vi "MainController5.vi"() -> ()   [LabVIEW 2014]
doc: "The top-level MainController VI for the RCM Control Stack application.\n\n\nMike Schultz (mschultz11711@gmail.com)"
uses:
  SRV VIs/SubVIs/SRV_Response Data Type.ctl
  SRV VIs/Motors/Motors Config/SRV_Motor Control Button Icons_TRUE.ctl
  SRV VIs/Motors/Motors Config/SRV_Motor Control Button Icons_FALSE.ctl
  SRV VIs/ImageProcessing/QR Code Detection Radio Buttons.ctl
  SRV VIs/SubVIs/SRV_SRV_Loops Notifier Methods.ctl
  SRV VIs/SRV_Main Controller Local Data.ctl
  SRV VIs/Motors/Motors Config/SRV_Motor Control Button Config.ctl
  SRV VIs/Motors/Motors Config/SRV_Motor Legos-Servo.ctl
  SRV VIs/Motors/Motors Config/SRV_Motor Control Commands Cluster.ctl
  SRV VIs/Motors/Motors Config/SRV_Motor Control Command Config.ctl
  SRV VIs/SubVIs/SRV_Streaming States.ctl
  SRV VIs/SubVIs/SRV_Streaming State.ctl
  SRV VIs/PacketMode/SRV_PM_Packet Mode Style.ctl
  SRV VIs/Support/SRV_Command-Data Queue Data Type.ctl
  SRV VIs/PacketMode/SRV_PM_Packet.ctl
  SRV VIs/Motors/SRV_Button Event Data.ctl
  SRV VIs/SubVIs/SRV_Streaming Modes.ctl
  <vilib>/Utility/miscctls.llb/LVBoundsTypeDef.ctl
  SRV VIs/ImageProcessing/QT_Image.ctl
  SRV VIs/SubVIs/SRV_Number of IMJ Requests Methods.ctl
  SRV VIs/SubVIs/SRVGlobals.vi
panel:
  in  "Window Enabled?":bool=TRUE
  out "Text.Scroll Position":u32
  in  "button E5":bool
  out "true E5":T1
  out "false E5":T2
  in  "button E4":bool
  out "true E4":T1
  out "false E4":T2
  in  "button E3":bool
  out "true E3":T1
  out "false E3":T2
  in  "button E1":bool
  out "true E1":T1
  out "false E1":T2
  in  "button E2":bool
  out "true E2":T1
  out "false E2":T2
  in  "button E7":bool
  out "true E7":T1
  out "false E7":T2
  in  "button E6":bool
  out "true E6":T1
  out "false E6":T2
  in  "button D7":bool
  out "true D7":T1
  out "false D7":T2
  in  "button A7":bool
  out "true A7":T1
  out "false A7":T2
  in  "button C7":bool
  out "true C7":T1
  out "false C7":T2
  in  "button B7":bool
  out "true B7":T1
  out "false B7":T2
  in  "button D6":bool
  out "true D6":T1
  out "false D6":T2
  in  "button A6":bool
  out "true A6":T1
  out "false A6":T2
  in  "button C6":bool
  out "true C6":T1
  out "false C6":T2
  in  "button B6":bool
  out "true B6":T1
  out "false B6":T2
  in  "button D5":bool
  out "true D5":T1
  out "false D5":T2
  in  "button A5":bool
  out "true A5":T1
  out "false A5":T2
  in  "button C5":bool
  out "true C5":T1
  out "false C5":T2
  in  "button B5":bool
  out "true B5":T1
  out "false B5":T2
  in  "button D4":bool
  out "true D4":T1
  out "false D4":T2
  in  "button A4":bool
  out "true A4":T1
  out "false A4":T2
  in  "button C4":bool
  out "true C4":T1
  out "false C4":T2
  in  "button B4":bool
  out "true B4":T1
  out "false B4":T2
  in  "button D3":bool
  out "true D3":T1
  out "false D3":T2
  in  "button A3":bool
  out "true A3":T1
  out "false A3":T2
  in  "button C3":bool
  out "true C3":T1
  out "false C3":T2
  in  "button B3":bool
  out "true B3":T1
  out "false B3":T2
  in  "button D2":bool
  out "true D2":T1
  out "false D2":T2
  in  "button A2":bool
  out "true A2":T1
  out "false A2":T2
  in  "button C2":bool
  out "true C2":T1
  out "false C2":T2
  in  "button B2":bool
  out "true B2":T1
  out "false B2":T2
  in  "Expand-Collapse":bool
  in  "button D1":bool
  out "true D1":T1
  out "false D1":T2
  in  "button A1":bool
  out "true A1":T1
  out "false A1":T2
  in  "button C1":bool
  out "true C1":T1
  out "false C1":T2
  in  "button B1":bool
  out "true B1":T1
  out "false B1":T2
  out "Overflow Indicator":bool
  out "ms Diff 3":u32
  out "ms Diff 2":u32
  out "ms Diff parse":u32
  out "ms Diff ##IMJ":u32
  out "ms Diff DQ":u32
  out "ms Diff":u32
  out "Response Data Type":T3=enum."No Data"
  out "i4":i32
  in  "Show Image":bool
  out "InPico State Change":bool
  in  "clear":bool
  out "Replies":string
  out "Number of IMJ Requests":i32
  out "XModem Replies":string[](array[string])
  out "i1":i32
  out "i2":i32
  out "Status":string
  out "The image":picture caption="new picture"
  out "IP Address":string
  out "In Pico":bool
  out "connected?":bool
  in  "Tab Control":T4(tab)=enum."Camera View"
  in  "Send Text":bool
  in  "ESC":bool
  in  "Direct Command to Send":string
  in  "Run CCode":bool
  in  "View Code":bool
  in  "Upload CCode":bool
  in  "C Code":string="int x,y,z;\nfor (x = 0; x < 2; x++) \n  {  \n    for (y = 0; y < 3; y++)\n       {       \n         for (z = 0; z < 2; z++)\n           {\n             printf(\"%d %d %d\\n\", x,y,z);   \n           }\n        } \n   }\nexit(1);"
  in  "load Text":bool
  in  "QR Code Detection":T5
  in  "Movie":bool
  in  "Camera":bool
  out "Cover":bool
  in  "Images Directory Path":path=path "C:/RCM_Images"
  out "YUV_SRV":cluster{"Y":sgl, "U":sgl, "V":sgl}
  in  "Plan":T6(radio)
  out "YUV_Calc":cluster{"Y":sgl, "U":sgl, "V":sgl}
  in  "Plan 2":T7(radio)
  in  "Plan 3":enum32{"Nothing", "Differencing"}(radio)
  in  "Plan 4":T8(radio)
  in  "Color to Send":string
  in  "Send Color":bool
  in  "vc Bins":T9(ring)=enum."Bin 2"
  in  "Show  Overlay":bool
  in  "Flip Image":bool
  in  "vz Bins":T10(ring)=enum."4 levels of U and 4 levels of V"
  in  "Threshold":i8(slide)=4 scale=1.0..9.0
  in  "firmware":path
  in  "Upload":bool
  in  "Version":bool
  in  "Edit Sensors Config":bool
  in  "Edit System Config":bool
  out "System Config":string
  in  "Edit Motors Config":bool
  in  "stop":bool
  # "Communication"
  # "Debug indicators below.\nA developer just needs to enlarge the decoration to include these at debug time."
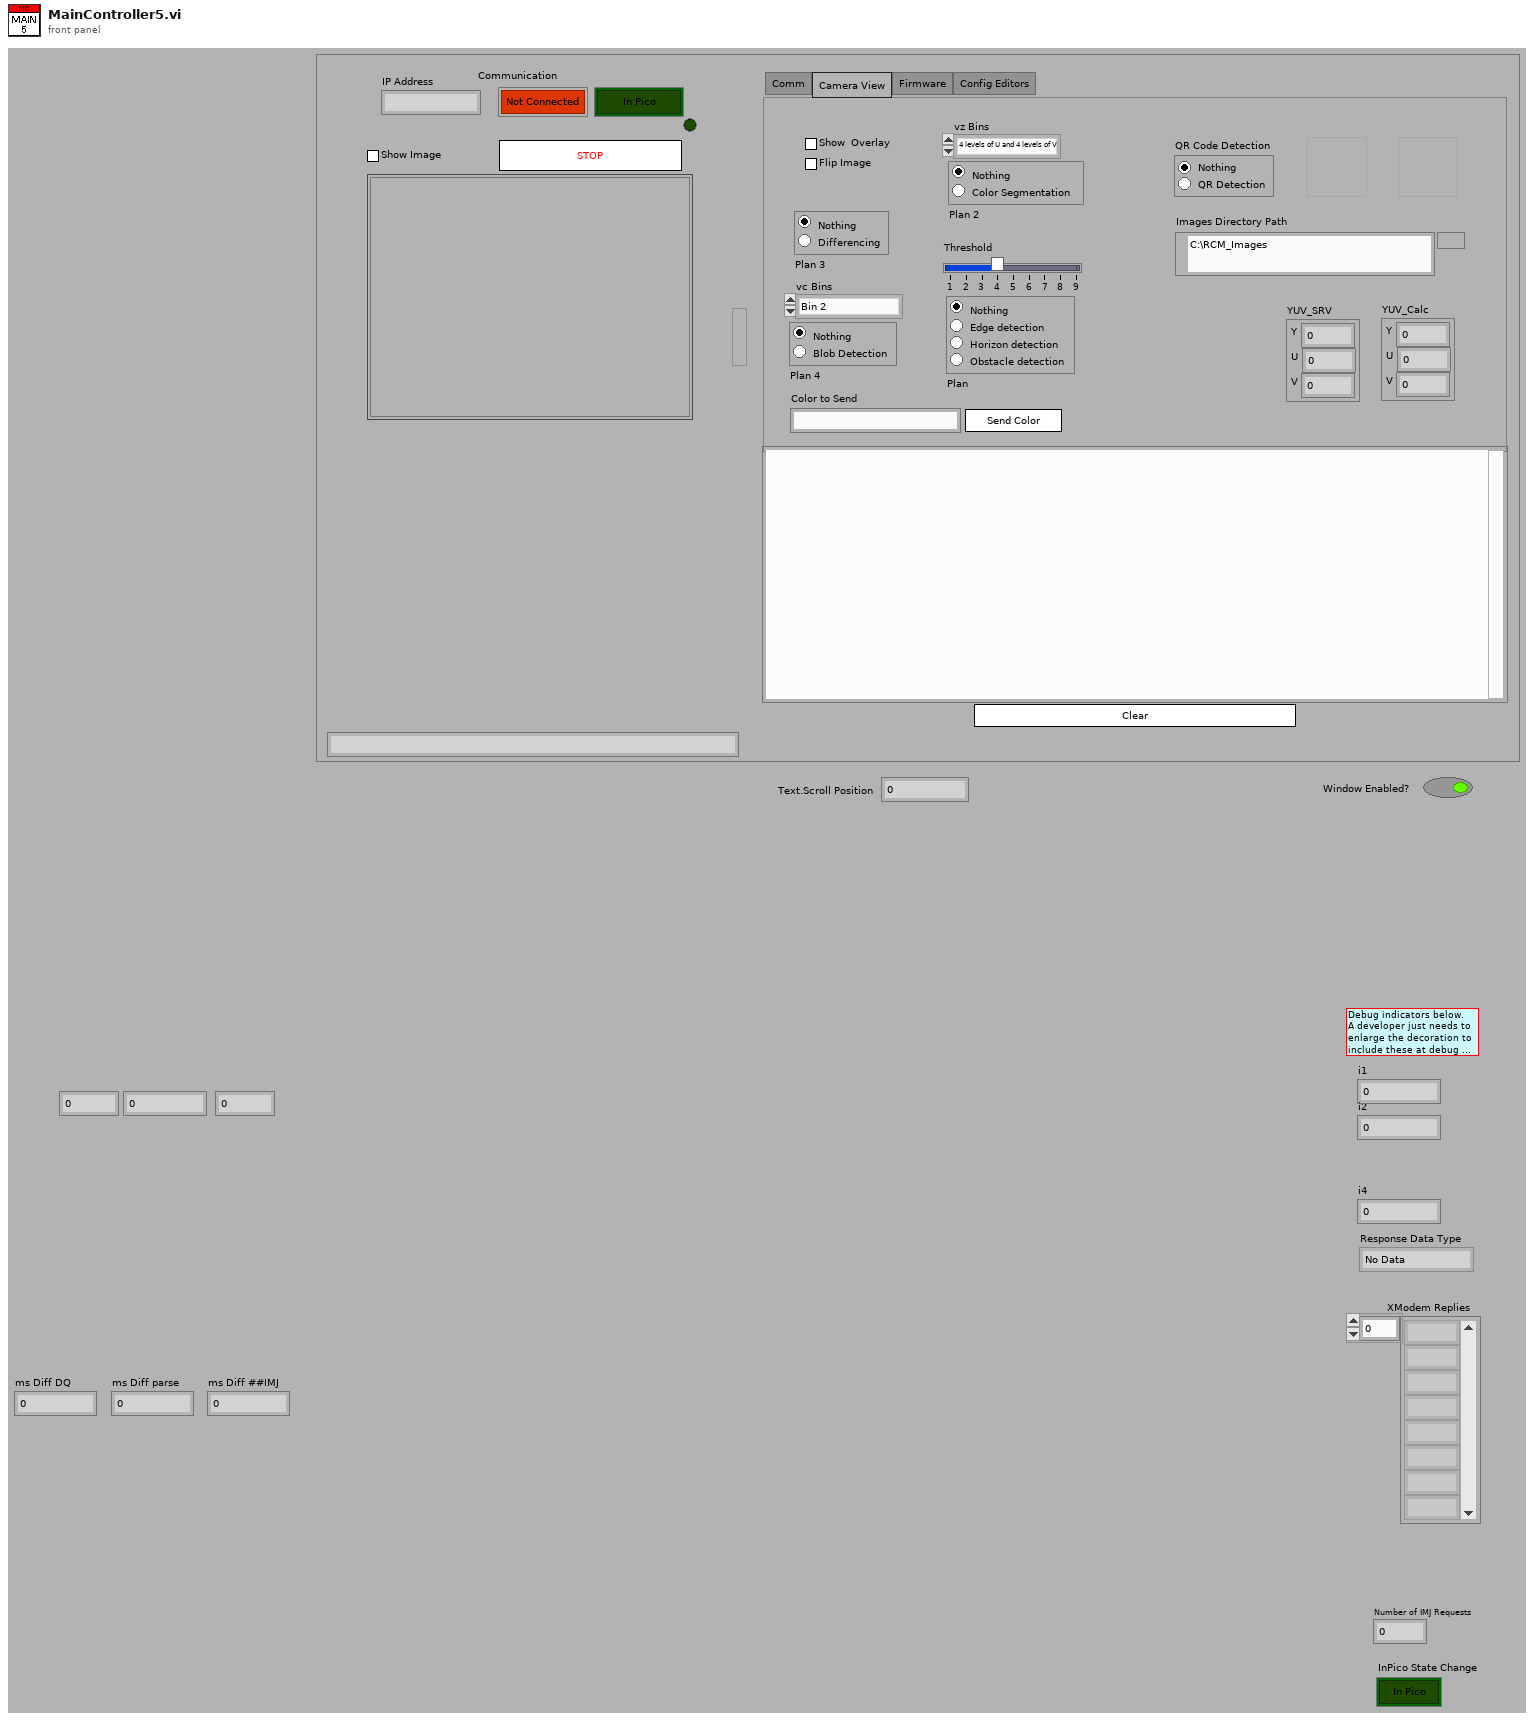
[diagram p1: front panel]
types:
  T1 = typedef "SRV_Motor Control Button Icons_TRUE.ctl" = u16
  T2 = typedef "SRV_Motor Control Button Icons_FALSE.ctl" = u16
  T3 = typedef "SRV_Response Data Type.ctl" = enum16{"Undefined Data", "##IMJ", "#B", "Leaving PicoC", "##vp", "##zZ", "##g:7", "##N$B", "##N$b", "##i$l", "##i$L", "##i$N", "##&NP,", "##&R,", "No Data"}
  T4 = enum32{"Comm", "Camera View", "Firmware", "Config Editors"}
  T5 = typedef "QR Code Detection Radio Buttons.ctl" = enum32{"Nothing", "QR Detection"}
  T6 = enum32{"Nothing", "Differencing", "Color Segmentation", "Edge detection", "Horizon detection", "Obstacle detection"}
  T7 = enum32{"Nothing", "Differencing", "Color Segmentation"}
  T8 = enum32{"Nothing", "Differencing", "Color Segmentation", "Edge detection", "Horizon detection", "Obstacle detection", "Blob Detection"}
  T9 = enum16{"Bin 0", "Bin 1", "Bin 2", "Bin 3", "Bin 4", "Bin 5", "Bin 6", "Bin 7", "Bin 9", "Bin 8", "Bin 10", "Bin 11", "Bin 12", "Bin 13", "Bin 14", "Bin 15"}
  T10 = enum16{"Zero all", "4 levels of Y, 2 levels of U, 2 levels of V", "4 levels of U and 4 levels of V", "even distribution across U and V", "16 grayscale levels"}
  T11 = typedef "SRV_Main Controller Local Data.ctl" = cluster{"user event":refnum<user-event>, "SRV":refnum<k5>, "Replies":refnum<vi>, "Status":refnum<vi>, "false refs":refnum<vi>[], "true refs":refnum<vi>[], "Motor Control Config":T12[], "Default Config Dir":path, "System Config Name":string, "Cached Streaming States":T16, "Main Controller ref":refnum<vi>, "Sensor View ref":refnum<vi>, "VISTA or Later?":bool, "button refs":refnum<vi>[]}
  T12 = typedef "SRV_Motor Control Button Config.ctl" = cluster{"Button Name":string, "Button Label":string, "Motor Type":T13, "Press Cmds":T14, "Release Cmds":T14, "Icon":T2}
  T13 = typedef "SRV_Motor Legos-Servo.ctl" = enum16{"Servo", "Legos", "Shared Var"}
  T14 = typedef "SRV_Motor Control Commands Cluster.ctl" = cluster{"Motor Control Commands Array":T15[]}
  T15 = typedef "SRV_Motor Control Command Config.ctl" = cluster{"I2C Address":u8, "Register":u8, "Value":u8, "Active":bool}
  T16 = typedef "SRV_Streaming States.ctl" = cluster{"Video":T17, "Sensors":T17}
  T17 = typedef "SRV_Streaming State.ctl" = cluster{"Enabled":bool, "Data":string}
  T18 = typedef "SRV_SRV_Loops Notifier Methods.ctl" = enum16{"Wait on Notification", "Send Notification", "Release Notifier"}
  T19 = typedef "SRV_PM_Packet.ctl" = cluster{"Packet Data":u8[], "Header Complete?":bool, "Complete?":bool, "Checksum OK?":bool, "Error?":bool}
  T20 = enum8{"Enabled", "Disabled", "Disabled and Grayed Out"}
  T21 = typedef "SRV_Command-Data Queue Data Type.ctl" = cluster{"Command":string, "Data":variant}
  T22 = typedef "SRV_PM_Packet Mode Style.ctl" = enum16{"Old", "New PM"}
  T23 = typedef "Semaphore RefNum" = refnum<k1>
  T24 = typedef "SRV_Button Event Data.ctl" = cluster{"Button NewVal":bool, "Button Index":i32}
  T25 = enum16{"Disable", "Frame Differencing", "Color Segmentation", "Edge Detection", "Horizon detection", "Obstacle detection", "Blob Detection", "Stereo processing"}
  T26 = typedef "SRV_Streaming Modes.ctl" = enum16{"Video", "Sensors"}
  T27 = typedef "LVBoundsTypeDef.ctl" = cluster{"Width":u32, "Height":u32}
  T28 = typedef "SRV_Number of IMJ Requests Methods.ctl" = enum16{"Read", "Increment", "Decrement", "Reset", "Close"}
  T29 = typedef "SRV_System Config.ctl" = cluster{"SRV IP Address":string, "Video Stream Rate Period (ms)":u32, "Enable Diagnostic Log":bool, "Watchdog 1 Config":T30, "Watchdog 2 Config":T30, "Sensor Window Filepath":path}
  T30 = typedef "SRV_Watchdog Config Cluster.ctl" = cluster{"Watchdog Name":string, "Watchdog Period (s)":dbl, "Watchdog Command":T15}
  T31 = typedef "QT_Image.ctl" = cluster{"Witdh":i32, "Height":i32, "Depth":i32, "data":u8[], "Compressed data":u8[], "Color table":u32[], "Duration":i32, "Options":i32, "Timestamp":i32, "ID":i32, "Reserved":i32, "Dialogs":u32}
  T32 = typedef "LVMouseTypeDef.ctl" = cluster{"Mouse Position":cluster{"X":i32, "Y":i32}, "Mouse Modifiers":cluster{"Button Down":bool, "Shift Mod":bool, "Menu Mod":bool, "Option Mod":bool}}
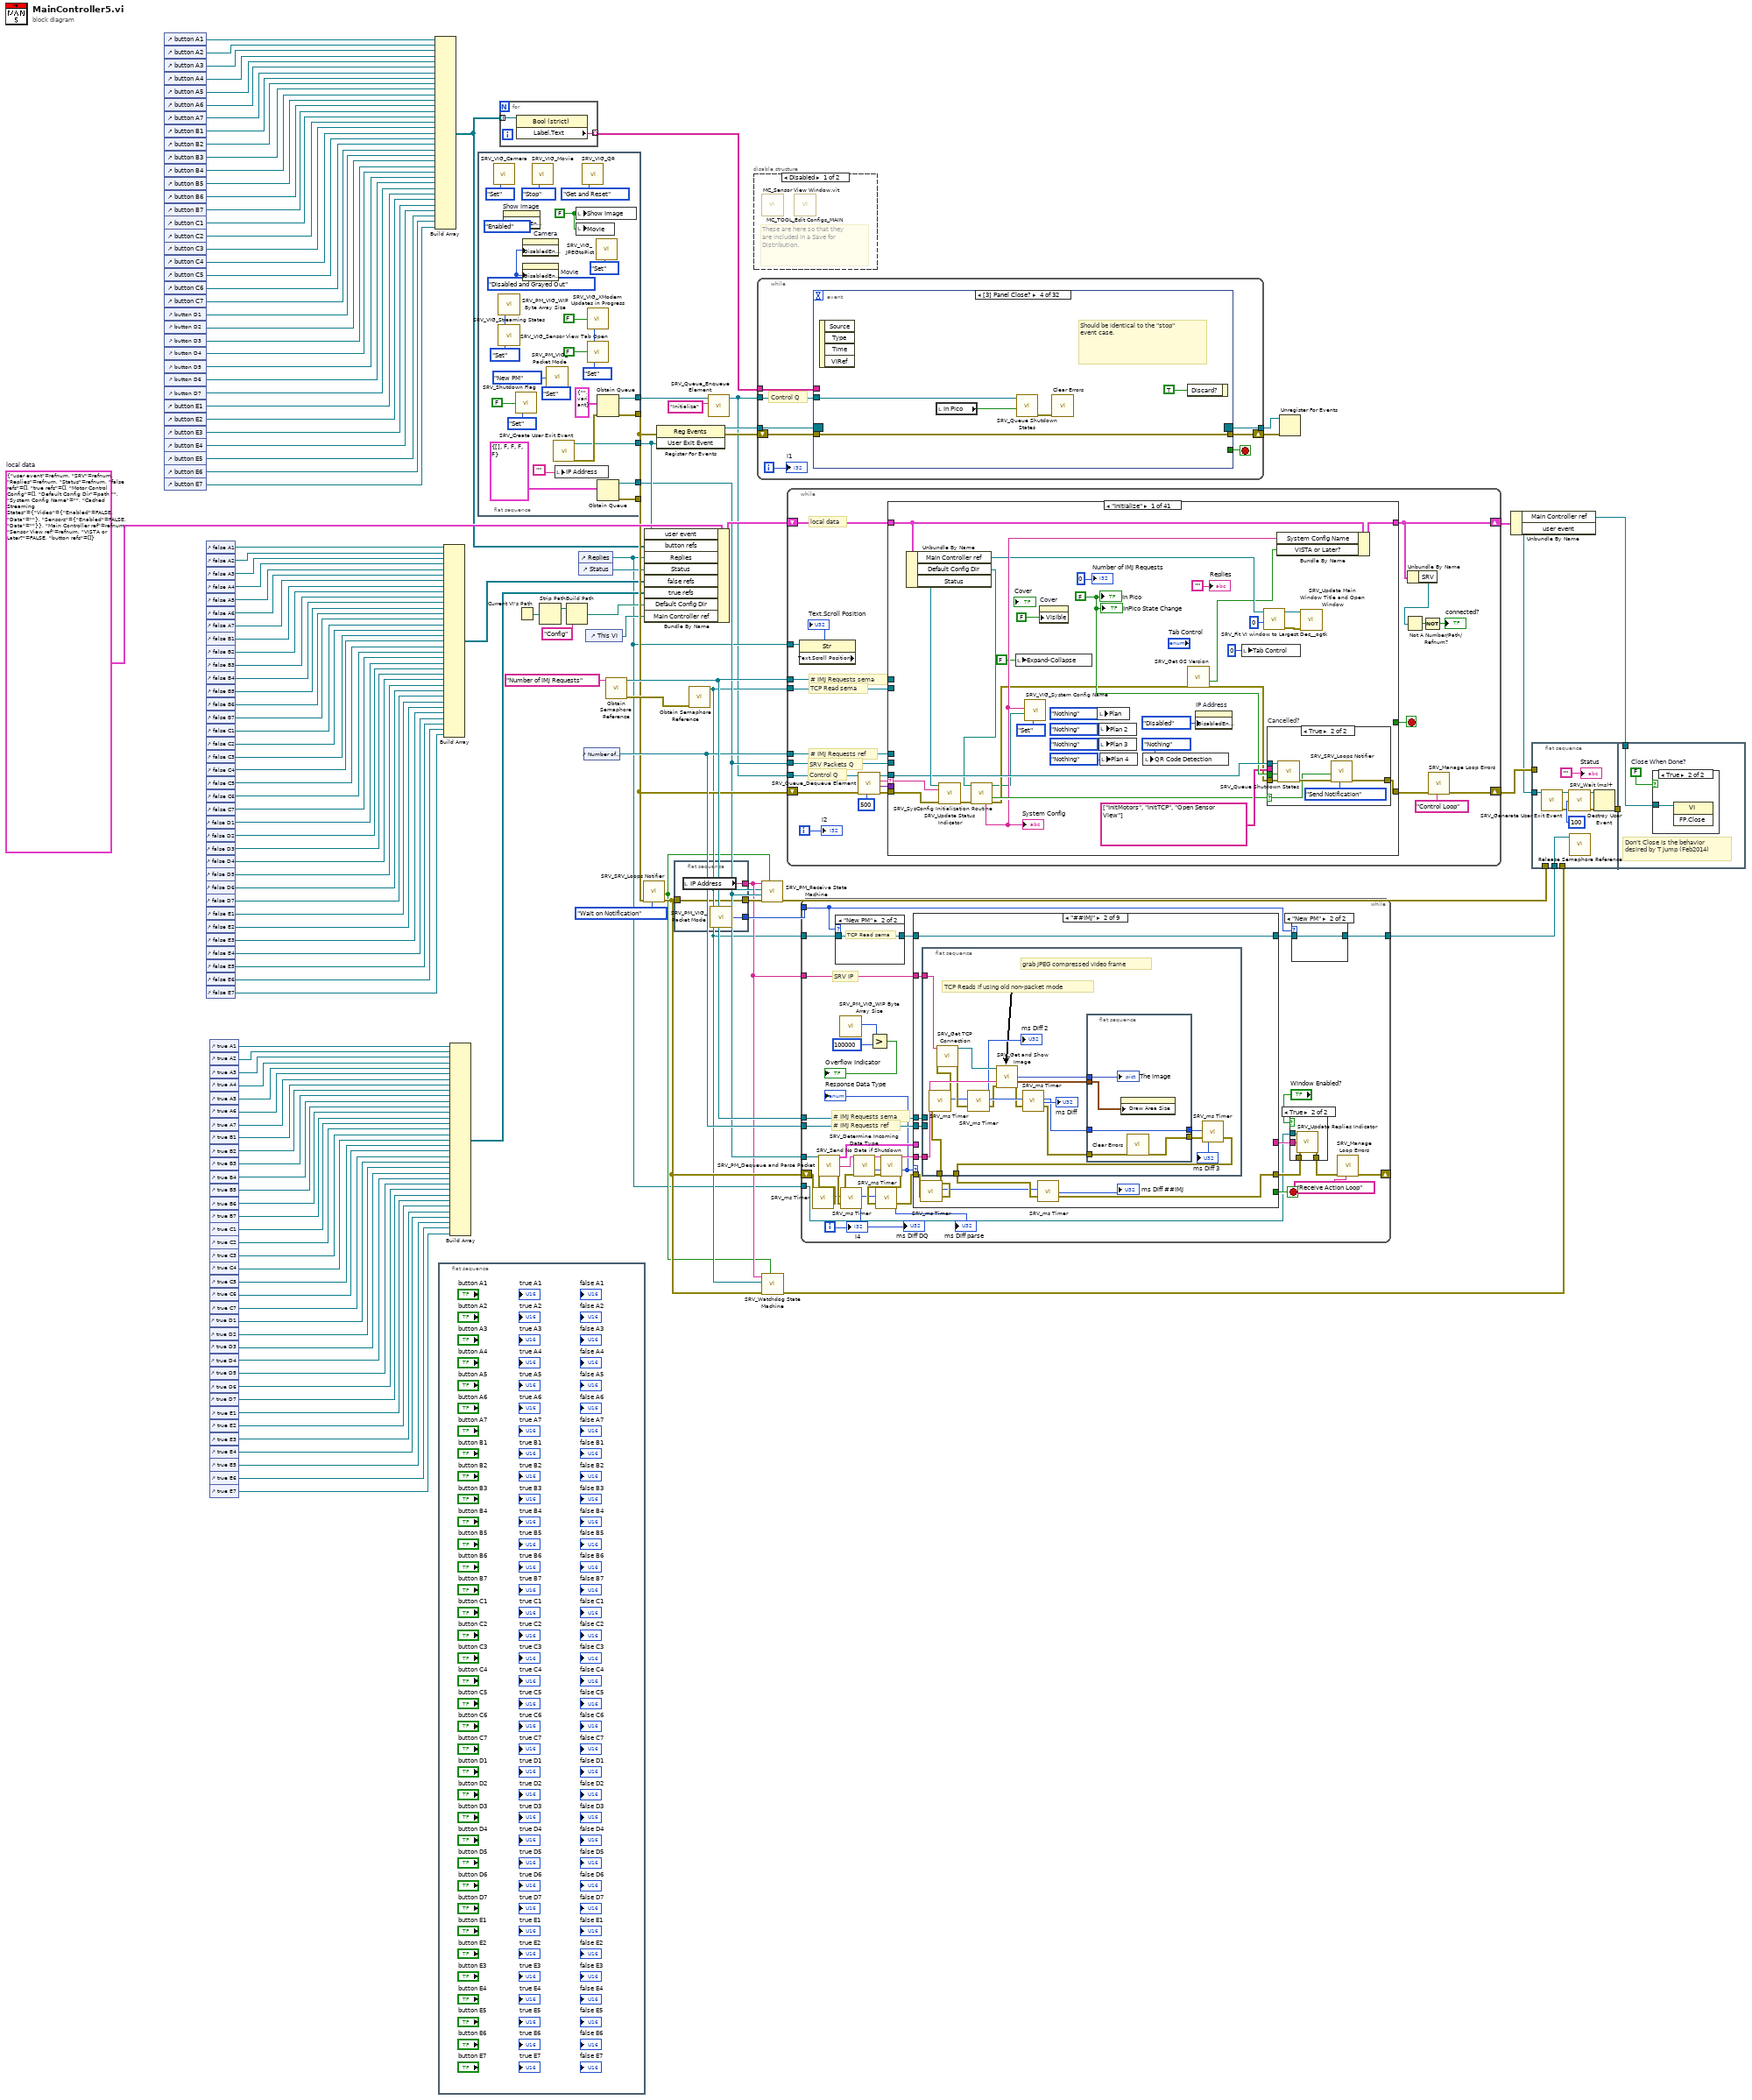
[diagram p0: block diagram]
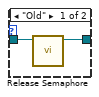
[diagram p5: hidden frame]
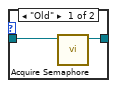
[diagram p6: hidden frame]
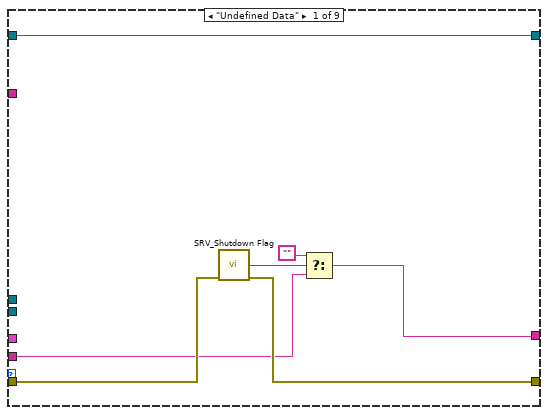
[diagram p7: hidden frame]
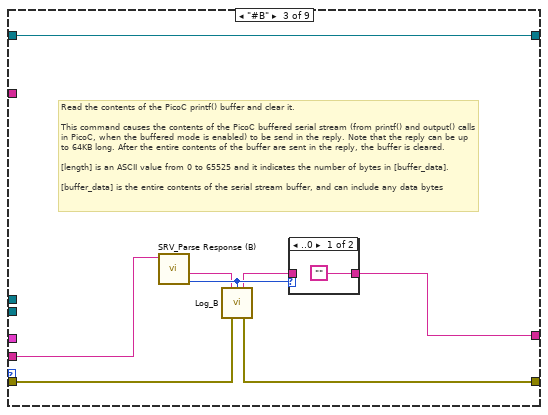
[diagram p8: hidden frame]
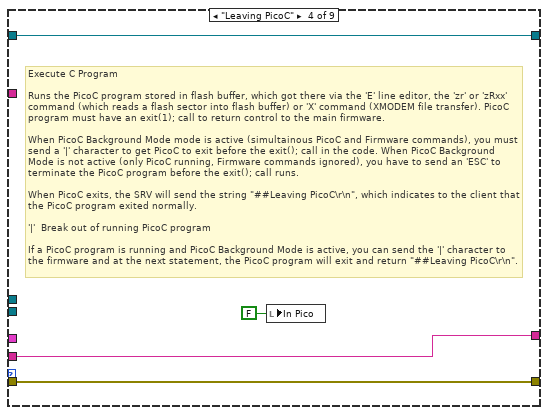
[diagram p10: hidden frame]
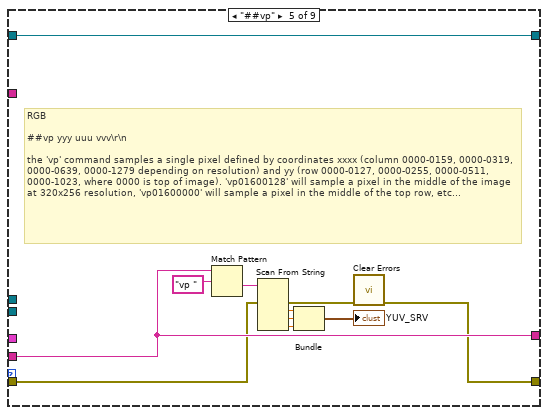
[diagram p11: hidden frame]
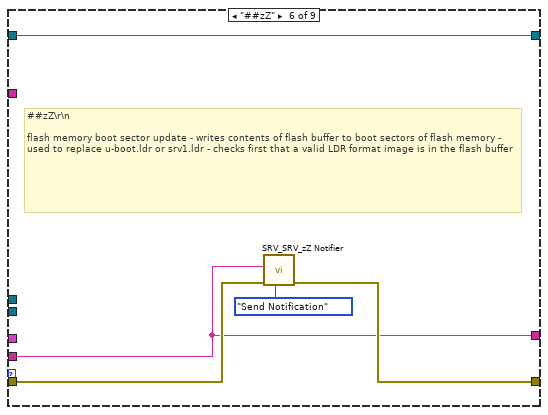
[diagram p12: hidden frame]
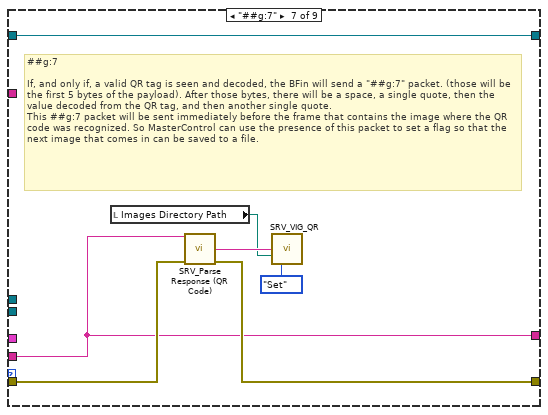
[diagram p13: hidden frame]
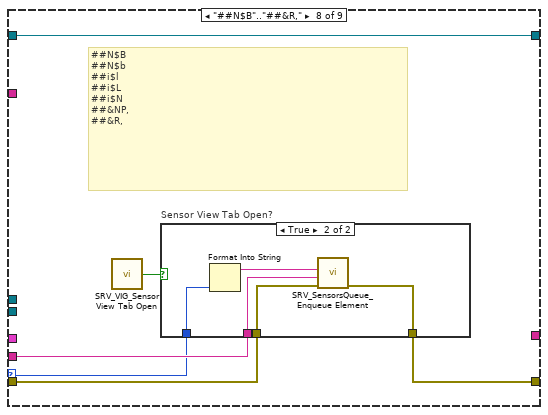
[diagram p14: hidden frame]
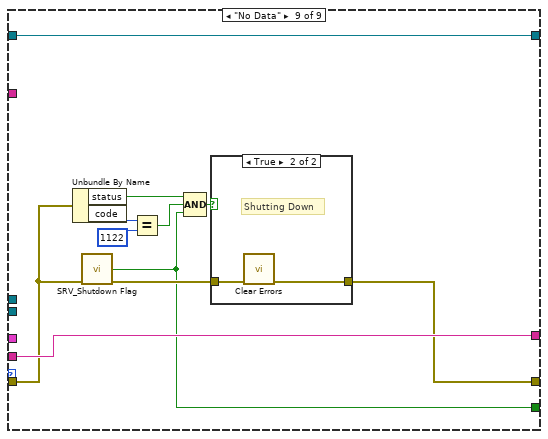
[diagram p16: hidden frame]
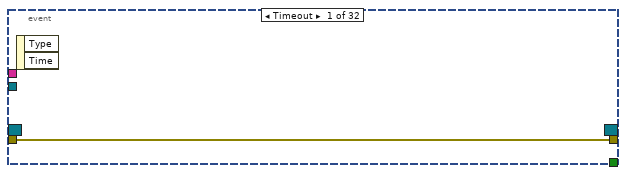
[diagram p18: hidden frame]
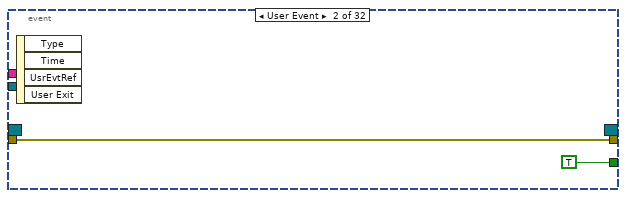
[diagram p19: hidden frame]
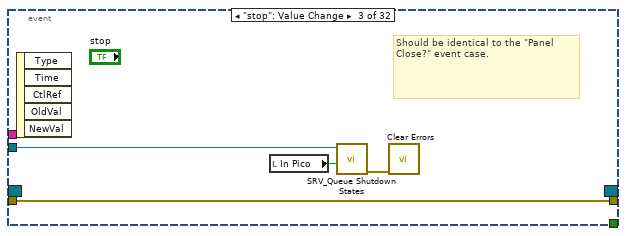
[diagram p20: hidden frame]
diagram:
  w136 = T11 {"user event"=refnum, "SRV"=refnum, "Replies"=refnum, "Status"=refnum, "false refs"=[], "true refs"=[], "Motor Control Config"=[], "Default Config Dir"=path "", "System Config Name"="", "Cached Streaming States"={"Video"={"Enabled"=FALSE, "Data"=""}, "Sensors"={"Enabled"=FALSE, "Data"=""}}, "Main Controller ref"=refnum, "Sensor View ref"=refnum, "VISTA or Later?"=FALSE, "button refs"=[]}  # local data
  n1 = control-ref of="button A1"() -> (w108:refnum<vi>)
  n2 = control-ref of="button A2"() -> (w107:refnum<vi>)
  n3 = control-ref of="button A3"() -> (w106:refnum<vi>)
  n4 = control-ref of="button A4"() -> (w105:refnum<vi>)
  n5 = control-ref of="button A5"() -> (w104:refnum<vi>)
  n6 = control-ref of="button A6"() -> (w103:refnum<vi>)
  n7 = control-ref of="button A7"() -> (w102:refnum<vi>)
  n8 = control-ref of="button B1"() -> (w101:refnum<vi>)
  n9 = control-ref of="button B2"() -> (w100:refnum<vi>)
  n10 = control-ref of="button B3"() -> (w99:refnum<vi>)
  n11 = control-ref of="button B4"() -> (w98:refnum<vi>)
  n12 = control-ref of="button B5"() -> (w97:refnum<vi>)
  n13 = control-ref of="button B6"() -> (w96:refnum<vi>)
  n14 = control-ref of="button B7"() -> (w95:refnum<vi>)
  n15 = control-ref of="button C1"() -> (w94:refnum<vi>)
  n16 = control-ref of="button C2"() -> (w93:refnum<vi>)
  n17 = control-ref of="button C3"() -> (w92:refnum<vi>)
  n18 = control-ref of="button C4"() -> (w91:refnum<vi>)
  n19 = control-ref of="button C5"() -> (w90:refnum<vi>)
  n20 = control-ref of="button C6"() -> (w89:refnum<vi>)
  n21 = control-ref of="button C7"() -> (w88:refnum<vi>)
  n22 = control-ref of="button D1"() -> (w87:refnum<vi>)
  n23 = control-ref of="button D2"() -> (w86:refnum<vi>)
  n24 = control-ref of="button D3"() -> (w85:refnum<vi>)
  n25 = control-ref of="button D4"() -> (w84:refnum<vi>)
  n26 = control-ref of="button D5"() -> (w83:refnum<vi>)
  n27 = control-ref of="button D6"() -> (w82:refnum<vi>)
  n28 = control-ref of="button D7"() -> (w81:refnum<vi>)
  n29 = control-ref of="button E1"() -> (w23:refnum<vi>)
  n30 = control-ref of="button E2"() -> (w22:refnum<vi>)
  n31 = control-ref of="button E3"() -> (w21:refnum<vi>)
  n32 = control-ref of="button E4"() -> (w20:refnum<vi>)
  n33 = control-ref of="button E5"() -> (w19:refnum<vi>)
  n34 = control-ref of="button E6"() -> (w18:refnum<vi>)
  n35 = control-ref of="button E7"() -> (w17:refnum<vi>)
  n36 = control-ref of="false A1"() -> (w52:refnum<vi>)
  n37 = control-ref of="false A2"() -> (w51:refnum<vi>)
  n38 = control-ref of="false A3"() -> (w50:refnum<vi>)
  n39 = control-ref of="false A4"() -> (w49:refnum<vi>)
  n40 = control-ref of="false A5"() -> (w48:refnum<vi>)
  n41 = control-ref of="false A6"() -> (w47:refnum<vi>)
  n42 = control-ref of="false A7"() -> (w46:refnum<vi>)
  n43 = control-ref of="false B1"() -> (w45:refnum<vi>)
  n44 = control-ref of="false B2"() -> (w44:refnum<vi>)
  n45 = control-ref of="false B3"() -> (w43:refnum<vi>)
  n46 = control-ref of="false B4"() -> (w42:refnum<vi>)
  n47 = control-ref of="false B5"() -> (w41:refnum<vi>)
  n48 = control-ref of="false B6"() -> (w40:refnum<vi>)
  n49 = control-ref of="false B7"() -> (w39:refnum<vi>)
  n50 = control-ref of="false C1"() -> (w38:refnum<vi>)
  n51 = control-ref of="false C2"() -> (w37:refnum<vi>)
  n52 = control-ref of="false C3"() -> (w36:refnum<vi>)
  n53 = control-ref of="false C4"() -> (w35:refnum<vi>)
  n54 = control-ref of="false C5"() -> (w34:refnum<vi>)
  n55 = control-ref of="false C6"() -> (w33:refnum<vi>)
  n56 = control-ref of="false C7"() -> (w32:refnum<vi>)
  n57 = control-ref of="false D1"() -> (w31:refnum<vi>)
  n58 = control-ref of="false D2"() -> (w30:refnum<vi>)
  n59 = control-ref of="false D3"() -> (w29:refnum<vi>)
  n60 = control-ref of="false D4"() -> (w28:refnum<vi>)
  n61 = control-ref of="false D5"() -> (w27:refnum<vi>)
  n62 = control-ref of="false D6"() -> (w26:refnum<vi>)
  n63 = control-ref of="false D7"() -> (w25:refnum<vi>)
  n64 = control-ref of="false E1"() -> (w9:refnum<vi>)
  n65 = control-ref of="false E2"() -> (w8:refnum<vi>)
  n66 = control-ref of="false E3"() -> (w7:refnum<vi>)
  n67 = control-ref of="false E4"() -> (w6:refnum<vi>)
  n68 = control-ref of="false E5"() -> (w5:refnum<vi>)
  n69 = control-ref of="false E6"() -> (w4:refnum<vi>)
  n70 = control-ref of="false E7"() -> (w3:refnum<vi>)
  n71 = control-ref of="true A1"() -> (w80:refnum<vi>)
  n72 = control-ref of="true A2"() -> (w79:refnum<vi>)
  n73 = control-ref of="true A3"() -> (w78:refnum<vi>)
  n74 = control-ref of="true A4"() -> (w77:refnum<vi>)
  n75 = control-ref of="true A5"() -> (w76:refnum<vi>)
  n76 = control-ref of="true A6"() -> (w75:refnum<vi>)
  n77 = control-ref of="true A7"() -> (w74:refnum<vi>)
  n78 = control-ref of="true B1"() -> (w73:refnum<vi>)
  n79 = control-ref of="true B2"() -> (w72:refnum<vi>)
  n80 = control-ref of="true B3"() -> (w71:refnum<vi>)
  n81 = control-ref of="true B4"() -> (w70:refnum<vi>)
  n82 = control-ref of="true B5"() -> (w69:refnum<vi>)
  n83 = control-ref of="true B6"() -> (w68:refnum<vi>)
  n84 = control-ref of="true B7"() -> (w67:refnum<vi>)
  n85 = control-ref of="true C1"() -> (w66:refnum<vi>)
  n86 = control-ref of="true C2"() -> (w65:refnum<vi>)
  n87 = control-ref of="true C3"() -> (w64:refnum<vi>)
  n88 = control-ref of="true C4"() -> (w63:refnum<vi>)
  n89 = control-ref of="true C5"() -> (w62:refnum<vi>)
  n90 = control-ref of="true C6"() -> (w61:refnum<vi>)
  n91 = control-ref of="true C7"() -> (w60:refnum<vi>)
  n92 = control-ref of="true D1"() -> (w59:refnum<vi>)
  n93 = control-ref of="true D2"() -> (w58:refnum<vi>)
  n94 = control-ref of="true D3"() -> (w57:refnum<vi>)
  n95 = control-ref of="true D4"() -> (w56:refnum<vi>)
  n96 = control-ref of="true D5"() -> (w55:refnum<vi>)
  n97 = control-ref of="true D6"() -> (w54:refnum<vi>)
  n98 = control-ref of="true D7"() -> (w53:refnum<vi>)
  n99 = control-ref of="true E1"() -> (w16:refnum<vi>)
  n100 = control-ref of="true E2"() -> (w15:refnum<vi>)
  n101 = control-ref of="true E3"() -> (w14:refnum<vi>)
  n102 = control-ref of="true E4"() -> (w13:refnum<vi>)
  n103 = control-ref of="true E5"() -> (w12:refnum<vi>)
  n104 = control-ref of="true E6"() -> (w11:refnum<vi>)
  n105 = control-ref of="true E7"() -> (w10:refnum<vi>)
  n106 = Build Array(w108, w107, w106, w105, w104, w103, w102, w101, w100, w99, w98, w97, w96, w95, w94, w93, w92, w91, w90, w89, w88, w87, w86, w85, w84, w83, w82, w81, w23, w22, w21, w20, w19, w18, w17) -> (w24:refnum<vi>[])
  n107 = flat-sequence {
    frame #0 {
    }
  }
  n108 = Build Array(w52, w51, w50, w49, w48, w47, w46, w45, w44, w43, w42, w41, w40, w39, w38, w37, w36, w35, w34, w33, w32, w31, w30, w29, w28, w27, w26, w25, w9, w8, w7, w6, w5, w4, w3) -> (w124:refnum<vi>[])
  n109 = Build Array(w80, w79, w78, w77, w76, w75, w74, w73, w72, w71, w70, w69, w68, w67, w66, w65, w64, w63, w62, w61, w60, w59, w58, w57, w56, w55, w54, w53, w16, w15, w14, w13, w12, w11, w10) -> (w123:refnum<vi>[])
  n110 = flat-sequence {
    tunnel: [w165] -> w137
    tunnel: [w166] -> w132
    tunnel: [w163] -> w133
    tunnel: [w159] -> w116
    tunnel: [w158] -> _
    frame #0 {
      w152 = T20."Disabled and Grayed Out" ("Disabled")
      w155 = enum16{"Get", "Set"}."Set" ("Method (Get)")
      w156 = enum16{"Get", "Set"}."Set" ("Method (Get)")
      w153 = FALSE ("Show Image")
      n111 = call "SRV_VIG_Camera.vi"("Method (Get)"=enum16{"Get", "Set"}."Set") -> ()  [unwired: 13 in, 2 out]
      n112 = call "SRV_PM_VIG_WIP Byte Array Size.vi"("Method (Get)"=w156) -> ()  [unwired: 9 in, 2 out]
      n113 = call "SRV_VIG_Streaming States.vi"("Method (Get)"=w156) -> ()  [unwired: 14 in, 1 out]
      n114 = property on="Show Image" class="Bool (strict)"("DisabledEnum"=T20."Enabled" ("Disabled")) -> ()  [unwired: 2 in, 2 out]
      n115 = call "SRV_Shutdown Flag.vi"("Shutdown Flag"=FALSE, "Method (Get)"=enum16{"Get", "Set"}."Set") -> ()  [unwired: 12 in, 2 out]
      n116 = property on="Camera" class="Bool"("DisabledEnum"=w152) -> ()  [unwired: 2 in, 2 out]
      n117 = property on="Movie" class="Bool (strict)"("DisabledEnum"=w152) -> ()  [unwired: 2 in, 2 out]
      n118 = call "SRV_VIG_Movie.vi"("Method (Get)"=enum16{"Get", "Start", "Stop"}."Stop") -> ()  [unwired: 11 in, 4 out]
      n119 = call "SRV_PM_VIG_Packet Mode.vi"("Packet Mode Style"=SRV_PM_Packet_Mode_Style."New PM", "Method (Get)"=enum16{"Get", "Set"}."Set") -> ()  [unwired: 13 in, 1 out]
      n120 = call "SRV_Create User Exit Event.vi"() -> ("error out"=w164:errorcluster, "User Exit Event"=w163:refnum<user-event>)  [unwired: 10 in]
      n121 = local write "IP Address"("") -> ()
      n122 = local write "Show Image"(w153) -> ()
      n123 = local write "Movie"(w153) -> ()
      n124 = call "SRV_VIG_QR.vi"("Method (Get and Reset)"=enum16{"Get and Reset", "Set"}."Get and Reset") -> ()  [unwired: 11 in, 4 out]
      n125 = call "SRV_VIG_XModem Updates in Progress.vi"("XModem Updates in Progress"=FALSE, "Method (Get)"=w155) -> ()  [unwired: 12 in, 2 out]
      n126 = call "SRV_VIG_Sensor View Tab Open.vi"("Sensor View Tab Open"=FALSE, "Method (Get)"=w155) -> ()  [unwired: 12 in, 2 out]
      n127 = call "SRV_VIG_JPEGtoPict.vi"("Method (Get)"=enum16{"Get", "Set"}."Set") -> ()  [unwired: 9 in, 2 out]
      n128 = Obtain Queue(element data type=T21 {"Command"="", "Data"=variant} ("Queue Data Type"), error in (no error)=w164) -> (queue out=w165:refnum<queue>, error out=w166:errorcluster)  [unwired: 3 in, 1 out]
      n129 = Obtain Queue(element data type=T19 {"Packet Data"=[], "Header Complete?"=FALSE, "Complete?"=FALSE, "Checksum OK?"=FALSE, "Error?"=FALSE} ("Packet")) -> (queue out=w159:refnum<queue>, error out=w158:errorcluster)  [unwired: 4 in, 1 out]
    }
  }
  n130 = for {
    tunnel: w24 -> [w173] mode=indexing
    tunnel: [w172] -> w122 mode=indexing
    n131 = property class="Bool (strict)"(reference=w173) -> ("Label.Text"=w172:string)  [unwired: 1 in, 2 out]
  }
  n132 = Current VI's Path() -> (path=w120:path)
  n133 = Strip Path(path=w120) -> (stripped path=w121:path)  [unwired: 1 out]
  n134 = Build Path(base path=w121, name or relative path="Config") -> (appended path=w118:path)
  n135 = control-ref of="Replies"() -> (w2:refnum<vi>)
  n136 = control-ref of="Status"() -> (w125:refnum<vi>)
  n137 = control-ref of="Number of IMJ Requests"() -> (w140:refnum<vi>)
  n138 = control-ref of="This VI"() -> (w115:refnum<vi>)
  n139 = call <vilib>:"Obtain Semaphore Reference.vi"("name (unnamed)"="Number of IMJ Requests") -> ("error out"=w144:errorcluster, "semaphore"=w141:T23)  [unwired: 4 in, 1 out]
  n140 = call "SRV_SRV_Loops Notifier.vi"("Notifier Methods"=SRV_SRV_Loops_Notifier_Methods."Wait on Notification", "error in (no error)"=w132) -> ("error out"=w113:errorcluster, "Cancelled?"=w110:bool)  [unwired: 8 in]
  n141 = Bundle By Name(cluster=w136, "user event"=w133, "button refs"=w24, "Replies"=w2, "Status"=w125, "false refs"=w124, "true refs"=w123, "Default Config Dir"=w118, "Main Controller ref"=w115) -> (w135:T11)
  n142 = register-events(error in=w132, w133) -> (reference out=w131:refnum<event-registration>, error out=w134:errorcluster)  [unwired: 1 in]
  n143 = flat-sequence {
    tunnel: [w176] -> w142
    tunnel: w113 -> [w176]
    tunnel: [w175] -> w112
    tunnel: [w174] -> w138
    frame #0 {
      n144 = local read "IP Address"() -> (w175:string)
      n145 = call "SRV_PM_VIG_Packet Mode.vi"() -> ("Packet Mode Style"=w174:T22)  [unwired: 15 in]
    }
  }
  n146 = call <vilib>:"Obtain Semaphore Reference.vi"("error in (no error)"=w144) -> ("semaphore"=w111:T23)  [unwired: 4 in, 2 out]
  n147 = call "SRV_Queue_Enqueue Element.vi"("Command"="Initialize" ("name (unnamed)"), "Command-Data Queue"=w137) -> ("Command-Data Queue out"=w1:refnum<queue>)  [unwired: 7 in, 2 out]
  n148 = disable-structure shown="Disabled" {
    frame Disabled {
      # "These are here so that they are included in a Save for Distribution."
      n149 = call "MC_Sensor View Window.vit"() -> ()  [unwired: 11 in, 1 out]
      n150 = call "MC_TOOL_Edit Configs_MAIN.vi"() -> ()  [unwired: 11 in, 1 out]
    }
    frame Enabled {
    }
  }
  n151 = while {
    tunnel: w1 -> [w184]
    shift-right: [w179] -> w130
    shift-left: w134 -> [w180]
    tunnel: w131 -> [w181]
    tunnel: [w178] -> w129
    tunnel: w122 -> [w177]
    i -> [w182]
    stop <- w183 stop-if-true
    # "Control Q"
    n152 = event shown="[3] Panel Close?" {
      selector: w181 -> [_ _ _ _ _ _ _ _ _ _ _ _ _ _ _ _ _ _ _ _ _ _ _ _ _ _ _ _ _ _ _ _]
      dyn-events: [_ _ _ _ _ _ _ _ _ _ _ _ _ _ _ _ _ _ _ _ _ _ _ _ _ _ _ _ _ _ _ _] -> w178
      timeout: _ -> [_ _ _ _ _ _ _ _ _ _ _ _ _ _ _ _ _ _ _ _ _ _ _ _ _ _ _ _ _ _ _ _]
      tunnel: w184 -> [_ _ w190 w194 w198 w201 w204 w208 w213 _ w228 w260 w271 w282 w293 w304 w315 w326 w337 w348 w359 w371 w378 w381 w384 w390 w394 w398 w402 w406 w410 w422]
      tunnel: [_ TRUE ("stop") _ _ _ _ _ _ _ _ _ _ _ _ _ _ _ _ _ _ _ _ _ _ _ _ _ _ _ _ _ _] -> w183
      tunnel: w180 -> [w185 w186 w188 w192 w197 w200 w203 w207 w212 w215 w227 w258 w266 w277 w288 w299 w310 w321 w332 w343 w354 w366 w377 w380 w383 w388 w392 w396 w400 w404 w408 w419]
      tunnel: [w185 w186 w188 w192 w197 w200 w203 w206 w211 w215 w227 w258 w266 w277 w288 w299 w310 w321 w332 w343 w354 w366 w377 w380 w383 w387 w391 w395 w399 w403 w407 w421] -> w179
      tunnel: w177 -> [_ _ _ _ _ _ _ _ _ _ _ _ _ _ _ _ _ _ _ _ _ _ _ _ _ _ _ _ _ _ _ w417]
      event Timeout {
        n153 = event-data() -> ()  [unwired: 1 in, 2 out]
      }
      event User Event {
        n154 = event-data() -> ()  [unwired: 1 in, 4 out]
      }
      event "stop": Value Change {
        # "Should be identical to the \"Panel Close?\" event case."
        n155 = event-data() -> ()  [unwired: 1 in, 5 out]
        n156 = local read "In Pico"() -> (w191:bool)
        n157 = call "SRV_Queue Shutdown States.vi"("In Pico"=w191, "Control Queue"=w190) -> ("error out"=w189:errorcluster)  [unwired: 8 in, 1 out]
        n158 = call <vilib>:"Clear Errors.vi"("error in (no error)"=w189) -> ()  [unwired: 5 in, 2 out]
      }
      event Panel Close? {
        # "Should be identical to the \"stop\" event case."
        n159 = event-data() -> ()  [unwired: 1 in, 4 out]
        n160 = local read "In Pico"() -> (w193:bool)
        n161 = call "SRV_Queue Shutdown States.vi"("In Pico"=w193, "Control Queue"=w194) -> ("error out"=w195:errorcluster)  [unwired: 8 in, 1 out]
        n162 = call <vilib>:"Clear Errors.vi"("error in (no error)"=w195) -> ()  [unwired: 5 in, 2 out]
        n163 = event-data("Discard?"=TRUE) -> ()  [unwired: 1 in, 1 out]
      }
      event "Send Text": Value Change {
        n164 = event-data() -> ()  [unwired: 1 in, 5 out]
        n165 = call "SRV_Queue_Enqueue Element.vi"("Command"="WriteSRV" ("name (unnamed)"), "Command-Data Queue"=w198) -> ()  [unwired: 7 in, 3 out]
      }
      event "Send Color": Value Change {
        n166 = event-data() -> ()  [unwired: 1 in, 5 out]
        n167 = call "SRV_Queue_Enqueue Element.vi"("Command"="WriteColor" ("name (unnamed)"), "Command-Data Queue"=w201) -> ()  [unwired: 7 in, 3 out]
      }
      event "The image": Mouse Up {
        n168 = event-data() -> ()  [unwired: 1 in, 1 out]
        n169 = call "SRV_Queue_Enqueue Element.vi"("Command"="RGB" ("name (unnamed)"), "Command-Data Queue"=w204) -> ()  [unwired: 7 in, 3 out]
      }
      event "Camera": Value Change {
        n170 = event-data() -> ()  [unwired: 1 in, 5 out]
        n171 = call "SRV_Queue_Enqueue Element.vi"("error in (no error)"=w207, "Command"="Camera" ("name (unnamed)"), "Command-Data Queue"=w208) -> ("error out"=w206:errorcluster)  [unwired: 6 in, 2 out]
      }
      event "Movie": Value Change {
        n172 = event-data() -> ("NewVal"=w210:bool)  [unwired: 1 in, 4 out]
        n173 = call "SRV_Queue_Enqueue Element.vi"("error in (no error)"=w212, "Data"=w210, "Command"="Movie" ("name (unnamed)"), "Command-Data Queue"=w213) -> ("error out"=w211:errorcluster)  [unwired: 5 in, 2 out]
      }
      event "load Text": Value Change {
        n174 = event-data() -> ()  [unwired: 1 in, 1 out]
        n175 = call "File Dialog2"("prompt"="Select a C code text file...", "pattern (all files)"="*.c;*.txt", "pattern label"="C Code Text File") -> ("selected path"=w216:path, "error out"=w217:errorcluster)  [unwired: 9 in, 2 out]
        n176 = case shown="No Error" w217 {
          selector: w217 -> [w222 _]
          tunnel: w216 -> [w221 _]
          frame No Error {
            n177 = Read from Text File(file (use dialog)=w221, error in=w222) -> (text=w223:string, error out=w224:errorcluster)  [unwired: 2 in, 2 out]
            n178 = case shown="No Error" w224 {
              tunnel: w223 -> [w225 _]
              frame No Error {
                n179 = local write "C Code"(w225) -> ()
              }
              frame Error {
              }
            }
          }
          frame Error {
          }
        }
      }
      event "Upload": Value Change {
        n180 = event-data() -> ()  [unwired: 1 in, 1 out]
        n181 = local read "firmware"() -> (w229:path)
        n182 = Empty String/Path?(string/path=w229) -> (empty?=w232:bool)
        n183 = case shown="True" w232 {
          tunnel: [FALSE ("cancelled") w250] -> w231
          tunnel: [w247 w249] -> w230
          tunnel: w229 -> [w247 _]
          frame False {
          }
          frame True {
            n184 = call "File Dialog3"("prompt"="Select a firmware file...", "pattern (all files)"="*.ldr", "pattern label"="Firmware File") -> ("selected path"=w249:path, "cancelled"=w250:bool, "error out"=w248:errorcluster)  [unwired: 9 in, 1 out]
            n185 = call <vilib>:"Clear Errors.vi"("error in (no error)"=w248) -> ()  [unwired: 5 in, 2 out]
          }
        }
        n186 = property on="Show Image" class="Bool (strict)"("DisabledEnum"=T20."Disabled and Grayed Out" ("Disabled")) -> ()  [unwired: 2 in, 2 out]
        n187 = case shown="False" w231 {
          tunnel: w228 -> [w238 _]
          tunnel: w230 -> [w236 _]
          frame False {
            n188 = flat-sequence {
              tunnel: [w239] -> w237
              tunnel: w236 -> [w240]
              frame #0 {
                n189 = local write "firmware"(w240) -> ()
                n190 = local read "In Pico"() -> (w239:bool)
              }
            }
            n191 = case shown="True" w237 {
              tunnel: w238 -> [w241 w244]
              tunnel: [w241 w243] -> w234
              tunnel: [_ w242] -> w233
              frame False {
              }
              frame True {
                n192 = call "SRV_Queue_Enqueue Element.vi"("Command"="Escape" ("name (unnamed)"), "Command-Data Queue"=w244) -> ("error out"=w242:errorcluster, "Command-Data Queue out"=w243:refnum<queue>)  [unwired: 7 in, 1 out]
              }
            }
            n193 = call "SRV_Queue Streaming Halt and Restore States.vi"("error in (no error)"=w233, "Commands"=T21[] [{"Command"="Upload", "Data"=variant}, {"Command"="Boot", "Data"=variant}], "Control Queue"=w234) -> ()  [unwired: 7 in, 2 out]
          }
          frame True {
          }
        }
      }
      event "Upload CCode": Value Change {
        n194 = event-data() -> ()  [unwired: 1 in, 1 out]
        n195 = local read "In Pico"() -> (w259:bool)
        n196 = case shown="True" w259 {
          tunnel: w260 -> [w261 w264]
          tunnel: [w261 w263] -> w257
          tunnel: [_ w262] -> w256
          frame False {
          }
          frame True {
            n197 = call "SRV_Queue_Enqueue Element.vi"("Command"="Escape" ("name (unnamed)"), "Command-Data Queue"=w264) -> ("error out"=w262:errorcluster, "Command-Data Queue out"=w263:refnum<queue>)  [unwired: 7 in, 1 out]
          }
        }
        n198 = call "SRV_Queue Streaming Halt and Restore States.vi"("error in (no error)"=w256, "Commands"=T21[] [{"Command"="CCode", "Data"=variant}], "Control Queue"=w257) -> ()  [unwired: 7 in, 2 out]
        n199 = property on="Show Image" class="Bool (strict)"("DisabledEnum"=T20."Disabled and Grayed Out" ("Disabled")) -> ()  [unwired: 2 in, 2 out]
      }
      event "Run CCode": Value Change {
        n200 = event-data() -> ()  [unwired: 1 in, 1 out]
        n201 = local read "In Pico"() -> (w268:bool)
        n202 = case shown="True" w268 {
          tunnel: w271 -> [w272 w275]
          tunnel: [w272 w274] -> w269
          tunnel: [_ w273] -> w267
          frame False {
          }
          frame True {
            n203 = call "SRV_Queue_Enqueue Element.vi"("Command"="Escape" ("name (unnamed)"), "Command-Data Queue"=w275) -> ("error out"=w273:errorcluster, "Command-Data Queue out"=w274:refnum<queue>)  [unwired: 7 in, 1 out]
          }
        }
        n204 = call "SRV_Queue_Enqueue Element.vi"("error in (no error)"=w267, "Command"="RunCode" ("name (unnamed)"), "Command-Data Queue"=w269) -> ()  [unwired: 6 in, 3 out]
      }
      event "View Code": Value Change {
        n205 = event-data() -> ()  [unwired: 1 in, 1 out]
        n206 = local read "In Pico"() -> (w279:bool)
        n207 = case shown="True" w279 {
          tunnel: w282 -> [w283 w286]
          tunnel: [w283 w285] -> w280
          tunnel: [_ w284] -> w278
          frame False {
          }
          frame True {
            n208 = call "SRV_Queue_Enqueue Element.vi"("Command"="Escape" ("name (unnamed)"), "Command-Data Queue"=w286) -> ("error out"=w284:errorcluster, "Command-Data Queue out"=w285:refnum<queue>)  [unwired: 7 in, 1 out]
          }
        }
        n209 = call "SRV_Queue_Enqueue Element.vi"("error in (no error)"=w278, "Command"="ViewCode" ("name (unnamed)"), "Command-Data Queue"=w280) -> ()  [unwired: 6 in, 3 out]
      }
      event "Plan": Value Change {
        n210 = event-data() -> ()  [unwired: 1 in, 1 out]
        n211 = local read "In Pico"() -> (w290:bool)
        n212 = case shown="True" w290 {
          tunnel: w293 -> [w294 w297]
          tunnel: [w294 w296] -> w291
          tunnel: [_ w295] -> w289
          frame False {
          }
          frame True {
            n213 = call "SRV_Queue_Enqueue Element.vi"("Command"="Escape" ("name (unnamed)"), "Command-Data Queue"=w297) -> ("error out"=w295:errorcluster, "Command-Data Queue out"=w296:refnum<queue>)  [unwired: 7 in, 1 out]
          }
        }
        n214 = call "SRV_Queue_Enqueue Element.vi"("error in (no error)"=w289, "Command"="EdgHorzObj Detection" ("name (unnamed)"), "Command-Data Queue"=w291) -> ()  [unwired: 6 in, 3 out]
      }
      event "Plan 2": Value Change {
        n215 = event-data() -> ()  [unwired: 1 in, 1 out]
        n216 = local read "In Pico"() -> (w301:bool)
        n217 = case shown="True" w301 {
          tunnel: w304 -> [w305 w308]
          tunnel: [w305 w307] -> w302
          tunnel: [_ w306] -> w300
          frame False {
          }
          frame True {
            n218 = call "SRV_Queue_Enqueue Element.vi"("Command"="Escape" ("name (unnamed)"), "Command-Data Queue"=w308) -> ("error out"=w306:errorcluster, "Command-Data Queue out"=w307:refnum<queue>)  [unwired: 7 in, 1 out]
          }
        }
        n219 = call "SRV_Queue_Enqueue Element.vi"("error in (no error)"=w300, "Command"="Color Segmentation" ("name (unnamed)"), "Command-Data Queue"=w302) -> ()  [unwired: 6 in, 3 out]
      }
      event "Plan 3": Value Change {
        n220 = event-data() -> ()  [unwired: 1 in, 1 out]
        n221 = local read "In Pico"() -> (w312:bool)
        n222 = case shown="True" w312 {
          tunnel: w315 -> [w316 w319]
          tunnel: [w316 w318] -> w313
          tunnel: [_ w317] -> w311
          frame False {
          }
          frame True {
            n223 = call "SRV_Queue_Enqueue Element.vi"("Command"="Escape" ("name (unnamed)"), "Command-Data Queue"=w319) -> ("error out"=w317:errorcluster, "Command-Data Queue out"=w318:refnum<queue>)  [unwired: 7 in, 1 out]
          }
        }
        n224 = call "SRV_Queue_Enqueue Element.vi"("error in (no error)"=w311, "Command"="Motion Detection_Differencing" ("name (unnamed)"), "Command-Data Queue"=w313) -> ()  [unwired: 6 in, 3 out]
      }
      event "Plan 4": Value Change {
        n225 = event-data() -> ()  [unwired: 1 in, 6 out]
        n226 = local read "In Pico"() -> (w323:bool)
        n227 = case shown="True" w323 {
          tunnel: w326 -> [w327 w330]
          tunnel: [w327 w329] -> w324
          tunnel: [_ w328] -> w322
          frame False {
          }
          frame True {
            n228 = call "SRV_Queue_Enqueue Element.vi"("Command"="Escape" ("name (unnamed)"), "Command-Data Queue"=w330) -> ("error out"=w328:errorcluster, "Command-Data Queue out"=w329:refnum<queue>)  [unwired: 7 in, 1 out]
          }
        }
        n229 = call "SRV_Queue_Enqueue Element.vi"("error in (no error)"=w322, "Command"="Motion Detection_Blobs" ("name (unnamed)"), "Command-Data Queue"=w324) -> ()  [unwired: 6 in, 3 out]
      }
      event "vz Bins": Value Change {
        n230 = event-data() -> ()  [unwired: 1 in, 6 out]
        n231 = local read "In Pico"() -> (w334:bool)
        n232 = case shown="True" w334 {
          tunnel: w337 -> [w338 w341]
          tunnel: [w338 w340] -> w335
          tunnel: [_ w339] -> w333
          frame False {
          }
          frame True {
            n233 = call "SRV_Queue_Enqueue Element.vi"("Command"="Escape" ("name (unnamed)"), "Command-Data Queue"=w341) -> ("error out"=w339:errorcluster, "Command-Data Queue out"=w340:refnum<queue>)  [unwired: 7 in, 1 out]
          }
        }
        n234 = call "SRV_Queue_Enqueue Element.vi"("error in (no error)"=w333, "Command"="Color Segmentation" ("name (unnamed)"), "Command-Data Queue"=w335) -> ()  [unwired: 6 in, 3 out]
      }
      event "vc Bins": Value Change {
        n235 = event-data() -> ()  [unwired: 1 in, 6 out]
        n236 = local read "In Pico"() -> (w345:bool)
        n237 = case shown="True" w345 {
          tunnel: w348 -> [w349 w352]
          tunnel: [w349 w351] -> w346
          tunnel: [_ w350] -> w344
          frame False {
          }
          frame True {
            n238 = call "SRV_Queue_Enqueue Element.vi"("Command"="Escape" ("name (unnamed)"), "Command-Data Queue"=w352) -> ("error out"=w350:errorcluster, "Command-Data Queue out"=w351:refnum<queue>)  [unwired: 7 in, 1 out]
          }
        }
        n239 = call "SRV_Queue_Enqueue Element.vi"("error in (no error)"=w344, "Command"="Blob Det_vc Bins" ("name (unnamed)"), "Command-Data Queue"=w346) -> ()  [unwired: 6 in, 3 out]
      }
      event "Threshold": Value Change {
        n240 = event-data() -> ()  [unwired: 1 in, 6 out]
        n241 = local read "In Pico"() -> (w356:bool)
        n242 = case shown="True" w356 {
          tunnel: w359 -> [w360 w363]
          tunnel: [w360 w362] -> w357
          tunnel: [_ w361] -> w355
          frame False {
          }
          frame True {
            n243 = call "SRV_Queue_Enqueue Element.vi"("Command"="Escape" ("name (unnamed)"), "Command-Data Queue"=w363) -> ("error out"=w361:errorcluster, "Command-Data Queue out"=w362:refnum<queue>)  [unwired: 7 in, 1 out]
          }
        }
        n244 = call "SRV_Queue_Enqueue Element.vi"("error in (no error)"=w355, "Command"="EdgHorzObj Detection" ("name (unnamed)"), "Command-Data Queue"=w357) -> ()  [unwired: 6 in, 3 out]
      }
      event Value Change {
        n245 = event-data() -> ("NewVal"=w365:T5)  [unwired: 1 in, 4 out]
        n246 = local read "In Pico"() -> (w368:bool)
        n247 = case shown="True" w368 {
          tunnel: w371 -> [w372 w375]
          tunnel: [w372 w374] -> w369
          tunnel: [_ w373] -> w367
          frame False {
          }
          frame True {
            n248 = call "SRV_Queue_Enqueue Element.vi"("Command"="Escape" ("name (unnamed)"), "Command-Data Queue"=w375) -> ("error out"=w373:errorcluster, "Command-Data Queue out"=w374:refnum<queue>)  [unwired: 7 in, 1 out]
          }
        }
        n249 = call "SRV_Queue_Enqueue Element.vi"("error in (no error)"=w367, "Data"=w365, "Command"="QR Code Detection" ("name (unnamed)"), "Command-Data Queue"=w369) -> ()  [unwired: 5 in, 3 out]
      }
      event "ESC": Value Change {
        n250 = event-data() -> ()  [unwired: 1 in, 1 out]
        n251 = call "SRV_Queue_Enqueue Element.vi"("Command"="Escape" ("name (unnamed)"), "Command-Data Queue"=w378) -> ()  [unwired: 7 in, 3 out]
      }
      event "Version": Value Change {
        n252 = event-data() -> ()  [unwired: 1 in, 1 out]
        n253 = call "SRV_Queue_Enqueue Element.vi"("Command"="Version" ("name (unnamed)"), "Command-Data Queue"=w381) -> ()  [unwired: 7 in, 3 out]
      }
      event "clear": Value Change {
        n254 = event-data() -> ()  [unwired: 1 in, 1 out]
        n255 = call "SRV_Queue_Enqueue Element.vi"("Command"="Clear" ("name (unnamed)"), "Command-Data Queue"=w384) -> ()  [unwired: 7 in, 3 out]
      }
      event "Show Image": Value Change {
        n256 = event-data() -> ()  [unwired: 1 in, 5 out]
        n257 = call "SRV_Queue_Enqueue Element.vi"("error in (no error)"=w388, "Data"="Show Image", "Command"="Video Streaming" ("element"), "Command-Data Queue"=w390) -> ("error out"=w387:errorcluster)  [unwired: 5 in, 2 out]
      }
      event "Show  Overlay": Value Change {
        n258 = event-data() -> ()  [unwired: 1 in, 6 out]
        n259 = call "SRV_Queue_Enqueue Element.vi"("error in (no error)"=w392, "Command"="GrabOverlay" ("name (unnamed)"), "Command-Data Queue"=w394) -> ("error out"=w391:errorcluster)  [unwired: 6 in, 2 out]
      }
      event "Flip Image": Value Change {
        n260 = event-data() -> ()  [unwired: 1 in, 6 out]
        n261 = call "SRV_Queue_Enqueue Element.vi"("error in (no error)"=w396, "Command"="FlipImage" ("name (unnamed)"), "Command-Data Queue"=w398) -> ("error out"=w395:errorcluster)  [unwired: 6 in, 2 out]
      }
      event "Edit Motors Config": Value Change {
        n262 = event-data() -> ()  [unwired: 1 in, 5 out]
        n263 = call "SRV_Queue_Enqueue Element.vi"("error in (no error)"=w400, "Command"="Edit Motors Config" ("name (unnamed)"), "Command-Data Queue"=w402) -> ("error out"=w399:errorcluster)  [unwired: 6 in, 2 out]
      }
      event "Edit Sensors Config": Value Change {
        n264 = event-data() -> ()  [unwired: 1 in, 5 out]
        n265 = call "SRV_Queue_Enqueue Element.vi"("error in (no error)"=w404, "Command"="Edit Sensors Config" ("name (unnamed)"), "Command-Data Queue"=w406) -> ("error out"=w403:errorcluster)  [unwired: 6 in, 2 out]
      }
      event "Edit System Config": Value Change {
        n266 = event-data() -> ()  [unwired: 1 in, 5 out]
        n267 = call "SRV_Queue_Enqueue Element.vi"("error in (no error)"=w408, "Command"="Edit System Config" ("name (unnamed)"), "Command-Data Queue"=w410) -> ("error out"=w407:errorcluster)  [unwired: 6 in, 2 out]
      }
      event "button A1", "button A2", "button A3", "button A4", "button A5", "button A6", "button A7", "button B1", "button B2", "button B3", "button B4", "button B5", "button B6", "button B7", "button C1", "button C2", "button C3", "button C4", "button C5", "button C6", "button C7", "button D1", "button D2", "button D3", "button D4", "button D5", "button D6", "button D7", "button E1", "button E2", "button E3", "button E4", "button E5", "button E6", "button E7": Value Change {
        n268 = event-data() -> ("NewVal"=w413:bool, "CtlRef"=w420:refnum<vi>)  [unwired: 1 in]
        n269 = property class="Bool (strict)"(reference=w420, error in=w419) -> (error out=w418:errorcluster, "Label.Text"=w416:string)  [unwired: 1 out]
        n270 = Search 1D Array(1D array=w417, element=w416) -> (index of element=w414:i32)  [unwired: 1 in]
        n271 = Bundle By Name(cluster=T24 {"Button NewVal"=FALSE, "Button Index"=-1} ("Button Event Data"), "Button NewVal"=w413, "Button Index"=w414) -> (w411:T24)
        n272 = call "SRV_Queue_Enqueue Element.vi"("error in (no error)"=w418, "Data"=w411, "Command"="Button Value Change" ("name (unnamed)"), "Command-Data Queue"=w422) -> ("error out"=w421:errorcluster)  [unwired: 5 in, 2 out]
      }
    }
    "i1" <- w182
  }
  n273 = call "SRV_PM_Receive State Machine.vi"("Cancelled?"=w110, "error in (no error)"=w142, "SRV_Packets queue"=w116, "TCP Read semaphore"=w111, "SRV IP Address"=w112) -> ("error out"=w128:errorcluster)  [unwired: 6 in]
  n274 = call "SRV_Watchdog State Machine.vi"("Cancelled?"=w110, "error in (no error)"=w113, "TCP Read semaphore"=w111, "SRV IP Address"=w112) -> ("error out"=w109:errorcluster)  [unwired: 7 in]
  n275 = while {
    tunnel: w1 -> [w439]
    shift-right: [w432] -> w139
    shift-left: w132 -> [w428]
    shift-right: [w430] -> w127
    shift-left: w135 -> [w445]
    tunnel: w111 -> [w441]
    tunnel: w140 -> [w436]
    tunnel: w141 -> [w433]
    tunnel: w116 -> [w425]
    tunnel: w2 -> [w424]
    i -> [w437]
    stop <- w442 stop-if-true
    # "SRV Packets Q"
    # "TCP Read sema"
    # "# IMJ Requests sema"
    # "# IMJ Requests ref"
    # "local data"
    # "Control Q"
    n276 = property class="Str"(reference=w424) -> ("Text.Scroll Position"=→"Text.Scroll Position":u32)  [unwired: 1 in, 2 out]
    n277 = call "SRV_Queue_Dequeue Element.vi"("timeout in ms (-1)"=500, "error in (no error)"=w428, "Command-Data Queue"=w439) -> ("error out"=w427:errorcluster, "Data"=w434:variant, "Command"=w435:string, "Command-Data Queue out"=w438:refnum<queue>)  [unwired: 3 in, 2 out]
    n278 = case shown="\"Initialize\"" w435 {
      selector: w435 -> [w475 _ w531 _ _ _ _ _ _ _ _ _ _ _ _ _ _ _ _ _ _ _ _ _ _ _ _ _ _ _ _ _ _ _ _ _ _ _ w1120 _ _]
      tunnel: [_ _ _ _ _ _ _ _ _ _ _ _ _ _ _ _ _ _ _ _ _ _ _ _ _ _ _ _ _ _ _ _ _ _ _ _ _ _ _ _ TRUE] -> w442
      tunnel: w434 -> [_ _ _ _ _ _ _ _ _ _ _ _ _ _ _ _ w769 _ _ _ _ _ _ w931 _ _ _ _ _ w997 _ _ _ _ w1081 _ _ _ _ _ _]
      tunnel: w438 -> [w466 _ w521 _ w620 w632 _ _ _ _ _ _ _ _ _ _ _ _ _ _ _ _ _ _ _ _ _ _ _ _ _ w1029 w1042 w1055 _ _ _ w1114 _ _ w1145]
      tunnel: w427 -> [w476 w504 w533 w583 w616 w622 w654 w665 w675 w690 w706 w722 w731 w738 w746 w752 w768 w790 w796 w819 w854 w911 w923 w933 w949 w960 w971 w981 w987 w996 w1013 w1033 w1046 w1059 w1080 w1096 w1107 w1113 w1117 w1128 w1152]
      tunnel: w445 -> [w464 w496 w518 w584 w618 w623 w650 w668 w678 w686 w702 w717 w724 w733 w740 w747 w759 w787 w791 w811 w844 w904 w920 w937 w946 w955 w968 w976 w990 w999 w1008 w1027 w1040 w1053 w1086 w1095 w1106 w1116 w1122 w1123 w1144]
      tunnel: [w463 w503 w522 w587 w618 w623 w650 w672 w682 w685 w701 w719 w726 w735 w742 w749 w771 w787 w793 w812 w846 w905 w921 w938 w947 w957 w969 w978 w990 w999 w1010 w1027 w1040 w1053 w1085 w1095 w1105 w1116 w1122 w1125 w1144] -> w430
      tunnel: w441 -> [_ _ _ _ _ _ _ _ _ _ _ _ _ _ _ _ _ _ _ w830 w867 w893 _ _ _ _ _ _ _ _ _ _ _ _ _ _ _ _ _ _ _]
      tunnel: w436 -> [_ _ _ _ _ _ w652 _ _ _ _ _ _ _ _ _ _ _ _ w821 w856 _ _ _ _ _ _ _ _ _ _ _ _ _ _ _ _ _ _ _ w1147]
      tunnel: w433 -> [_ _ _ _ _ _ w651 _ _ _ _ _ _ _ _ _ _ _ _ w816 w850 _ _ _ _ _ _ _ _ _ _ _ _ _ _ _ _ _ _ _ w1148]
      tunnel: [w465 w499 w527 w589 w619 w633 w648 w673 w683 w689 w705 w721 w728 w737 w745 w751 w772 w789 w795 w829 w851 w899 w916 w936 w939 w959 w965 w980 w986 w993 w1012 w1030 w1043 w1056 w1082 w1092 w1107 w1110 w1119 w1127 w1136] -> w426
      tunnel: w425 -> [_ _ _ _ _ _ _ _ _ _ _ _ _ _ _ _ _ _ _ _ _ _ _ _ _ _ _ _ _ _ _ _ _ _ _ _ _ _ _ _ w1140]
      frame "Initialize" {
        w462 = FALSE ("In Pico")
        n279 = Unbundle By Name(w464) -> ("Main Controller ref"=w455:refnum<vi>, "Default Config Dir"=w459:path, "Status"=w467:refnum<vi>)
        n280 = call "SRV_Update Status Indicator.vi"("Status ref"=w467, "Status"=w475, "error in (no error)"=w476) -> ("error out"=w460:errorcluster)  [unwired: 11 in, 1 out]
        n281 = call "SRV_SysConfig Initialization Routine.vi"("Config Dir"=w459, "error in (no error)"=w460) -> ("SystemConfig Filepath"=w451:path, "Cancelled?"=w458:bool, "Sys Config Name"=w457:string, "error out"=w453:errorcluster)  [unwired: 8 in, 2 out]
        "System Config" <- w457
        n282 = local write "Expand-Collapse"(FALSE ("Expand-Collapse")) -> ()
        n283 = call "SRV_VIG_System Config Name.vi"("Method (Get)"=enum16{"Get", "Set"}."Set", "SystemConfig Filepath"=w451, "System Config Name"=w457) -> ()  [unwired: 6 in, 3 out]
        n284 = property on="Cover" class="Bool (strict)"("Visible"=FALSE) -> ()  [unwired: 2 in, 2 out]
        n285 = local write "Plan"(T6."Nothing" ("Plan")) -> ()
        n286 = local write "Plan 2"(T7."Nothing" ("Plan")) -> ()
        n287 = local write "Plan 3"(enum32{"Nothing", "Differencing"}."Nothing" ("Plan")) -> ()
        n288 = local write "Plan 4"(T8."Nothing" ("Plan")) -> ()
        n289 = local write "QR Code Detection"(QR_Code_Detection_Radio_Buttons."Nothing" ("QR Code Detection")) -> ()
        n290 = call "SRV_Get OS Version.vi"("error in (no error)"=w453) -> ("Equal or Newer Version?"=w454:bool, "error out"=w452:errorcluster)  [unwired: 12 in, 1 out]
        n291 = property on="IP Address" class="Str"("DisabledEnum"=T20."Disabled" ("Disabled")) -> ()  [unwired: 2 in, 2 out]
        n292 = local write "Tab Control"(u32 0) -> ()
        n293 = call "SRV_Fit VI window to Largest Dec__ogtk.vi"("border spacing (2 px)"=0, "VI Ref (calling VI)"=w455) -> ("error out"=w472:errorcluster, "dup VI Ref"=w473:refnum<vi>)  [unwired: 4 in]
        n294 = case "Cancelled?" shown="True" w458 {
          selector: w458 -> [_ w487]
          tunnel: w466 -> [w482 w492]
          tunnel: [w481 w488] -> w465
          tunnel: w452 -> [w480 w493]
          tunnel: w462 -> [_ w491]
          tunnel: string[] ["InitMotors", "InitTCP", "Open Sensor View"] -> [w479 _]
          frame False {
            n295 = for {
              tunnel: w482 -> [w486]
              shift-right: [w485] -> w481
              shift-left: w480 -> [w484]
              tunnel: w479 -> [w483] mode=indexing
              n296 = call "SRV_Queue_Enqueue Element.vi"("error in (no error)"=w484, "Command"=w483, "Command-Data Queue"=w486) -> ("error out"=w485:errorcluster)  [unwired: 6 in, 2 out]
            }
          }
          frame True {
            n297 = call "SRV_Queue Shutdown States.vi"("error in (no error)"=w493, "In Pico"=w491, "Control Queue"=w492) -> ("error out"=w489:errorcluster)  [unwired: 7 in, 1 out]
            n298 = call "SRV_SRV_Loops Notifier.vi"("Notifier Methods"=SRV_SRV_Loops_Notifier_Methods."Send Notification", "error in (no error)"=w489, "Cancelled? (F)"=w487) -> ("error out"=w488:errorcluster)  [unwired: 7 in, 1 out]
          }
        }
        n299 = Bundle By Name(cluster=w464, "System Config Name"=w457, "VISTA or Later?"=w454) -> (w463:T11)
        n300 = call "SRV_Update Main Window Title and Open Window.vi"("VI ref"=w473, "error in (no error)"=w472) -> ()  [unwired: 12 in, 2 out]
        "Number of IMJ Requests" <- 0 ("Number of IMJ Requests")
        "In Pico" <- w462
        "Replies" <- ""
        "InPico State Change" <- w462
      }
      frame "InitMotors" {
        n301 = call "SRV_Main Config Paths.vi"("local data"=w496) -> ("local data dup"=w495:T11, "MotorsConfig Filepath"=w497:path)  [unwired: 8 in, 5 out]
        n302 = Unbundle By Name(w495) -> ("button refs"=w494:refnum<vi>[], "false refs"=w501:refnum<vi>[], "true refs"=w500:refnum<vi>[])
        n303 = call "SRV_Check File Exists with Dialog.vi"("Filepath"=w497, "File Type"="Motor Config File", "error in (no error)"=w504) -> ("Filepath dup"=w505:path, "File Exists?"=w498:bool, "error out"=w506:errorcluster)  [unwired: 10 in]
        n304 = call "SRV_Initialize Motor Buttons.vi"("Motors Config File Path"=w505, "button refs"=w494, "false refs"=w501, "true refs"=w500, "Init from File (F)"=w498, "error in (no error)"=w506) -> ("Motor Control Config"=w502:T12[], "error out"=w499:errorcluster)  [unwired: 8 in]
        n305 = Bundle By Name(cluster=w496, "Motor Control Config"=w502) -> (w503:T11)
      }
      frame "InitTCP" {
        n306 = Unbundle By Name(w518) -> ("Status"=w532:refnum<vi>)
        n307 = call "SRV_Main Config Paths.vi"("local data"=w518) -> ("SystemConfig Filepath"=w517:path)  [unwired: 8 in, 6 out]
        n308 = call "SRV_Update Status Indicator.vi"("Status ref"=w532, "Status"=w531, "error in (no error)"=w533) -> ("Status ref out"=w519:refnum<vi>, "error out"=w515:errorcluster)  [unwired: 11 in]
        n309 = call "SRV_Read System Config File.vi"("System Config File Path"=w517, "error in (no error)"=w515) -> ("System Config"=w516:T29, "error out"=w514:errorcluster)  [unwired: 10 in, 2 out]
        n310 = call "SRV_Init_TCP Comm Loop.vi"("error in (no error)"=w514, "System Config File Path in"=w517) -> ("error out"=w525:errorcluster, "Cancelled?"=w511:bool, "SRV IP Address out"=w524:string, "connection ID"=w526:refnum<k5>)  [unwired: 6 in]
        n311 = Unbundle By Name(w516) -> ("Enable Diagnostic Log"=w513:bool)
        n312 = case "Cancelled?" shown="False" w511 {
          tunnel: w526 -> [w546 w565]
          tunnel: w525 -> [w545 w566]
          tunnel: [w544 w565] -> w510
          tunnel: [w543 w566] -> w523
          frame False {
            n313 = call "SRV_PM_VIG_Packet Mode.vi"() -> ("Packet Mode Style"=w542:T22)  [unwired: 15 in]
            n314 = case shown="\"New PM\"" w542 {
              tunnel: w546 -> [w554 w562]
              tunnel: w545 -> [w553 w563]
              tunnel: [w552 w559] -> w544
              tunnel: [w551 w558] -> w543
              frame "Old" {
                n315 = call "CameraSetup.vi"("error in (no error)"=w553, "Task"=T25."Disable", "SRV In"=w554) -> ("error out"=w549:errorcluster, "SRV Out"=w548:refnum<k5>)  [unwired: 7 in]
                n316 = call "SRV_Write_Comm.vi"("error in (no error)"=w549, "Command Sent"="V", "SRV In"=w548) -> ("error out"=w551:errorcluster, "SRV Out"=w552:refnum<k5>)  [unwired: 6 in, 1 out]
              }
              frame "New PM" {
                n317 = call "SRV_PM_App Initialization Routine.vi"("Packet Mode Enable (T)"=TRUE, "Read Response (F)"=FALSE, "error in (no error)"=w563, "timeout ms (25,000)"=5000, "connection ID"=w562) -> ("error out"=w557:errorcluster, "connection ID out"=w560:refnum<k5>)  [unwired: 3 in, 2 out]
                n318 = call "CameraSetup.vi"("error in (no error)"=w557, "Task"=T25."Disable", "SRV In"=w560) -> ("error out"=w558:errorcluster, "SRV Out"=w559:refnum<k5>)  [unwired: 7 in]
              }
            }
          }
          frame True {
          }
        }
        n319 = flat-sequence {
          tunnel: w513 -> [w540]
          tunnel: [SRV_SRV_Loops_Notifier_Methods."Send Notification" ("Notifier Methods")] -> w512
          frame #0 {
            n320 = call "SRV_VIG_System Config-Enable Diagnostic Logging.vi"("Enable Diagnostic Log"=w540, "Method (Get)"=enum16{"Get", "Set"}."Set") -> ()  [unwired: 13 in, 1 out]
          }
        }
        n321 = flat-sequence {
          tunnel: w524 -> [w567]
          tunnel: w523 -> [w568]
          tunnel: [w568] -> w520
          frame #0 {
            "IP Address" <- w567
          }
        }
        n322 = call "SRV_Update Status Indicator.vi"("Status ref"=w519, "error in (no error)"=w520) -> ("error out"=w530:errorcluster)  [unwired: 12 in, 1 out]
        n323 = case "Cancelled?" shown="False" w511 {
          selector: w511 -> [w576 w579]
          tunnel: w530 -> [w573 w582]
          tunnel: [w575 w581] -> w529
          tunnel: w521 -> [w574 w580]
          tunnel: [w576 w579] -> w528
          tunnel: w510 -> [w571 w577]
          tunnel: [w570 w577] -> w509
          tunnel: [w569 _] -> w508
          frame False {
            n324 = local read "In Pico"() -> (w572:bool)
            n325 = call "SRV_Error 56 Dialog.vi"("SRV In"=w571, "error in (no error)"=w573, "In Pico"=w572, "Control Queue"=w574) -> ("error out"=w575:errorcluster, "Retry?"=w569:bool, "SRV Out"=w570:refnum<k5>)  [unwired: 4 in, 1 out]
          }
          frame True {
            n326 = local read "In Pico"() -> (w578:bool)
            n327 = call "SRV_Queue Shutdown States.vi"("error in (no error)"=w582, "In Pico"=w578, "Control Queue"=w580) -> ("error out"=w581:errorcluster)  [unwired: 7 in, 1 out]
          }
        }
        n328 = case "Retry?" shown="False" w508 {
          tunnel: w529 -> [w537 w538]
          tunnel: w528 -> [w536 _]
          tunnel: [w535 w538] -> w527
          tunnel: w512 -> [w534 _]
          frame False {
            n329 = call "SRV_SRV_Loops Notifier.vi"("Notifier Methods"=w534, "error in (no error)"=w537, "Cancelled? (F)"=w536) -> ("error out"=w535:errorcluster)  [unwired: 7 in, 1 out]
          }
          frame True {
          }
        }
        n330 = Bundle By Name(cluster=w518, "SRV"=w509) -> (w522:T11)
      }
      frame "Open Sensor View" {
        n331 = call "SRV_Shutdown Flag.vi"() -> ("Shutdown Flag out"=w585:bool)  [unwired: 14 in, 1 out]
        n332 = case "Shutdown Flag set?" shown="False" w585 {
          tunnel: [w602 _] -> w588
          tunnel: [w601 _] -> w586
          tunnel: w584 -> [w594 _]
          frame False {
            n333 = Unbundle By Name(w594) -> ("SRV"=w597:refnum<k5>, "VISTA or Later?"=w592:bool, "Main Controller ref"=w590:refnum<vi>)
            n334 = call "SRV_Main Config Paths.vi"("local data"=w594) -> ("SystemConfig Filepath"=w593:path, "SensorsConfig Filepath"=w598:path)  [unwired: 8 in, 5 out]
            n335 = local read "Expand-Collapse"() -> (w591:bool)
            n336 = call "SRV_Get Sensor Window Filepath.vi"("System Config File Path"=w593) -> ("error out"=w595:errorcluster, "Sensor Window Filepath"=w596:path)  [unwired: 9 in]
            n337 = call "SRV_Update Streaming States VIG.vi"("Enabled"=TRUE, "Streaming Modes"=SRV_Streaming_Modes."Sensors") -> ()  [unwired: 14 in]
            n338 = call "SRV_Launch Sensor View Tab GUI.vi"("VI Path"=w596, "Sensors Config File Path"=w598, "SRV In"=w597, "Vista or Later?"=w592, "error in (no error)"=w595, "Main Controller ref"=w590, "Expand-Collapse"=w591) -> ("VI refnum out"=w601:refnum<vi>, "error out"=w602:errorcluster)  [unwired: 6 in, 1 out]
          }
          frame True {
          }
        }
        n339 = Bundle By Name(cluster=w584, "Sensor View ref"=w586) -> (w587:T11)
        n340 = Select(t=w583, s=w583, f=w588) -> (s? t:f=w589:errorcluster)
      }
      frame "" {
        n341 = Unbundle By Name(w618) -> ("Status"=w610:refnum<vi>, "VISTA or Later?"=w603:bool, "Sensor View ref"=w617:refnum<vi>, "Main Controller ref"=w615:refnum<vi>)
        n342 = call "SRV_Manage Window Sizes.vi"("Sensor View ref"=w617, "Vista or Later?"=w603, "Main Controller ref"=w615, "Expand-Collapse"="Expand-Collapse", "error in (no error)"=w616) -> ("error out"=w614:errorcluster)  [unwired: 10 in]
        n343 = Select(t="Collapse to hide tabs..." ("Tip Strip"), s="Expand-Collapse", f="Expand to show tabs..." ("Tip Strip")) -> (s? t:f=w613:string)
        n344 = Select(t=T27 {"Width"=1180, "Height"=25} ("Size"), s="Expand-Collapse", f=T27 {"Width"=412, "Height"=25} ("Size")) -> (s? t:f=w608:T27)
        n345 = property on="Expand-Collapse" class="Bool (strict)"(error in=w614, "TipStrip"=w613) -> (error out=w606:errorcluster)  [unwired: 1 in, 1 out]
        n346 = property class="Str"(reference=w610, error in=w606, "Size"=w608) -> (error out=w605:errorcluster)  [unwired: 1 out]
        n347 = call "SRV_Queue_Enqueue Element.vi"("error in (no error)"=w605, "Command"="Manage InPico State" ("element"), "Command-Data Queue"=w620) -> ("error out"=w619:errorcluster)  [unwired: 6 in, 2 out]
      }
      frame "Manage InPico State" {
        # "The boolean logic here is all about getting one more PicoC Buffer Read after the In Pico light goes off."
        n348 = local read "InPico State Change"() -> (w629:bool)
        n349 = local read "In Pico"() -> (w626:bool)
        n350 = call "SRV_In PicoC State Change.vi"("In Pico"=w626, "InPico State Change"=w629) -> ("Read PicoC Buffer?"=w624:bool, "InPico State Change out"=w628:bool)  [unwired: 8 in]
        n351 = call "SRV_Manage Time Interval for Read.vi"("Some State"=w626, "Read Interval (1000 ms)"=u32 100) -> ("Time to Read?"=w631:bool, "State Change?"=w627:bool)  [unwired: 12 in]
        n352 = Compound Arithmetic op=OR(w624, w626, w627) -> (w625:bool)
        n353 = local write "InPico State Change"(w628) -> ()
        n354 = case shown="True" w625 {
          tunnel: w622 -> [w634 w641]
          tunnel: [w634 w640] -> w633
          tunnel: w632 -> [_ w639]
          tunnel: w631 -> [_ w637]
          tunnel: w627 -> [_ w638]
          tunnel: w624 -> [_ w636]
          frame False {
          }
          frame True {
            n355 = Compound Arithmetic op=OR(w636, w637, w638) -> (w635:bool)
            n356 = case shown="True" w635 {
              tunnel: w641 -> [w642 w646]
              tunnel: [w642 w645] -> w640
              tunnel: w639 -> [_ w644]
              frame False {
              }
              frame True {
                n357 = call "SRV_Queue_Enqueue Element.vi"("error in (no error)"=w646, "Command"="Read PicoC Buffer", "Command-Data Queue"=w644) -> ("error out"=w645:errorcluster)  [unwired: 6 in, 2 out]
              }
            }
          }
        }
      }
      frame "GrabImage" {
        w647 = FALSE  # Show Image
        n358 = Unbundle By Name(w650) -> ("SRV"=w649:refnum<k5>)
        n359 = Not(x=w647) -> (.not. x?=w653:bool)
        n360 = property on="Cover" class="Bool (strict)"("Visible"=w653) -> ()  [unwired: 2 in, 2 out]
        n361 = case shown="True" w647 {
          tunnel: w654 -> [w655 w660]
          tunnel: [w655 w662] -> w648
          tunnel: w649 -> [_ w661]
          tunnel: w652 -> [_ w658]
          tunnel: w651 -> [_ w656]
          frame False {
          }
          frame True {
            n362 = call "SRV_Number of IMJ Requests Methods.vi"("Number of IMJ Requests ref"=w658, "semaphore ref"=w656, "error in (no error)"=w660, "Number of IMJ Requests Methods (Read)"=SRV_Number_of_IMJ_Requests_Methods."Increment" ("Number of IMJ Requests Methods")) -> ("error out"=w659:errorcluster)  [unwired: 7 in, 4 out]
            n363 = call "SRV_Write_Comm.vi"("error in (no error)"=w659, "Command Sent"="I", "SRV In"=w661) -> ("error out"=w662:errorcluster)  [unwired: 6 in, 2 out]
          }
        }
      }
      frame "GrabOverlay" {
        w669 = "O"  # Turn Overlay Off
        w670 = "o"  # Turn Overlay On
        n364 = Unbundle By Name(w668) -> ("SRV"=w666:refnum<k5>)
        n365 = Select(t=w670, s="Show  Overlay", f=w669) -> (s? t:f=w667:string)
        n366 = call "SRV_Write_Comm.vi"("error in (no error)"=w665, "Command Sent"=w667, "SRV In"=w666) -> ("error out"=w673:errorcluster, "SRV Out"=w671:refnum<k5>)  [unwired: 6 in, 1 out]
        n367 = Bundle By Name(cluster=w668, "SRV"=w671) -> (w672:T11)
      }
      frame "FlipImage" {
        w679 = "Y"  # FlipImage Off
        w680 = "y"  # FlipImage On
        n368 = Unbundle By Name(w678) -> ("SRV"=w676:refnum<k5>)
        n369 = Select(t=w680, s="Flip Image", f=w679) -> (s? t:f=w677:string)
        n370 = call "SRV_Write_Comm.vi"("error in (no error)"=w675, "Command Sent"=w677, "SRV In"=w676) -> ("error out"=w683:errorcluster, "SRV Out"=w681:refnum<k5>)  [unwired: 6 in, 1 out]
        n371 = Bundle By Name(cluster=w678, "SRV"=w681) -> (w682:T11)
      }
      frame "WriteSRV" {
        n372 = Unbundle By Name(w686) -> ("SRV"=w687:refnum<k5>)
        n373 = case shown="Default" "Direct Command to Send" {
          selector: "Direct Command to Send" -> [_ w693]
          tunnel: w687 -> [w691 w698]
          tunnel: [w691 w697] -> w684
          tunnel: w690 -> [w692 w696]
          tunnel: [w692 w695] -> w689
          frame "" {
          }
          frame Default {
            n374 = call "SRV_Write_Comm.vi"("error in (no error)"=w696, "Command Sent"=w693, "SRV In"=w698) -> ("error out"=w695:errorcluster, "Command Sent dup"=w694:string, "SRV Out"=w697:refnum<k5>)  [unwired: 6 in]
            n375 = case shown="\"!\", \"Q\"" w694 {
              frame Default {
              }
              frame "!", "Q" {
                w699 = TRUE ("In Pico")
                n376 = local write "InPico State Change"(w699) -> ()
                n377 = local write "In Pico"(w699) -> ()
              }
            }
          }
        }
        n378 = Bundle By Name(cluster=w686, "SRV"=w684) -> (w685:T11)
      }
      frame "WriteColor" {
        n379 = Unbundle By Name(w702) -> ("SRV"=w703:refnum<k5>)
        n380 = case shown="Default" "Color to Send" {
          selector: "Color to Send" -> [_ w709]
          tunnel: w703 -> [w707 w714]
          tunnel: [w707 w713] -> w700
          tunnel: w706 -> [w708 w712]
          tunnel: [w708 w711] -> w705
          frame "" {
          }
          frame Default {
            n381 = call "SRV_Write_Comm.vi"("error in (no error)"=w712, "Command Sent"=w709, "SRV In"=w714) -> ("error out"=w711:errorcluster, "Command Sent dup"=w710:string, "SRV Out"=w713:refnum<k5>)  [unwired: 6 in]
            n382 = case shown="\"!\", \"Q\"" w710 {
              frame Default {
              }
              frame "!", "Q" {
                w715 = TRUE ("In Pico")
                n383 = local write "InPico State Change"(w715) -> ()
                n384 = local write "In Pico"(w715) -> ()
              }
            }
          }
        }
        n385 = Bundle By Name(cluster=w702, "SRV"=w700) -> (w701:T11)
      }
      frame "RunCode" {
        w720 = TRUE ("In Pico")
        n386 = Unbundle By Name(w717) -> ("SRV"=w718:refnum<k5>)
        n387 = call "SRV_Write_Comm.vi"("error in (no error)"=w722, "Command Sent"="Q" ("name (unnamed)"), "SRV In"=w718) -> ("error out"=w721:errorcluster, "SRV Out"=w716:refnum<k5>)  [unwired: 6 in, 1 out]
        n388 = local write "In Pico"(w720) -> ()
        n389 = local write "InPico State Change"(w720) -> ()
        n390 = Bundle By Name(cluster=w717, "SRV"=w716) -> (w719:T11)
      }
      frame "ViewCode" {
        # "Wait here to avoid enqueuing more \"I\" (Grab Image) before this has a chance to read all the code in the lower loop. Without waiting, you get binary jpeg info along with the read code in the Replies window.\n\nThis is not an elegant solution...should code semaphore type functionality but what is trickier than with the XModem code is the verification that you are done reading the C code comes in the lower loop.\n\nIs there some sort of term char that goes with the message that we can read until we find??"
        n391 = Unbundle By Name(w724) -> ("SRV"=w727:refnum<k5>)
        n392 = call "SRV_Write_Comm.vi"("error in (no error)"=w731, "Command Sent"="zd" ("name (unnamed)"), "SRV In"=w727) -> ("error out"=w729:errorcluster, "SRV Out"=w725:refnum<k5>)  [unwired: 6 in, 1 out]
        n393 = call "SRV_Wait (ms)+.vi"("milliseconds to wait"=u32 500 ("Delay (ms)"), "error in (no error)"=w729) -> ("error out"=w728:errorcluster)  [unwired: 12 in, 1 out]
        n394 = Bundle By Name(cluster=w724, "SRV"=w725) -> (w726:T11)
      }
      frame "Escape" {
        w739 = FALSE ("Enable?")
        n395 = Unbundle By Name(w733) -> ("SRV"=w736:refnum<k5>)
        n396 = local write "In Pico"(w739) -> ()
        n397 = call "PicoC_Mode.vi"("error in (no error)"=w738, "Enable?"=w739, "SRV In"=w736) -> ("error out"=w737:errorcluster, "SRV Out"=w734:refnum<k5>)  [unwired: 7 in]
        n398 = Bundle By Name(cluster=w733, "SRV"=w734) -> (w735:T11)
      }
      frame "GoPico" {
        w744 = TRUE ("Enable?")
        # "Never gets here."
        n399 = Unbundle By Name(w740) -> ("SRV"=w743:refnum<k5>)
        n400 = local write "In Pico"(w744) -> ()
        n401 = local write "InPico State Change"(w744) -> ()
        n402 = call "PicoC_Mode.vi"("error in (no error)"=w746, "Enable?"=w744, "SRV In"=w743) -> ("error out"=w745:errorcluster, "SRV Out"=w741:refnum<k5>)  [unwired: 7 in]
        n403 = Bundle By Name(cluster=w740, "SRV"=w741) -> (w742:T11)
      }
      frame "Version" {
        n404 = Unbundle By Name(w747) -> ("SRV"=w750:refnum<k5>)
        n405 = call "SRV_Write_Comm.vi"("error in (no error)"=w752, "Command Sent"="V", "SRV In"=w750) -> ("error out"=w751:errorcluster, "SRV Out"=w748:refnum<k5>)  [unwired: 6 in, 1 out]
        n406 = Bundle By Name(cluster=w747, "SRV"=w748) -> (w749:T11)
      }
      frame "Video Streaming" {
        w765 = "$v2"  # Turn Video Streaming Off
        w766 = "$v1"  # Turn Video Streaming On
        n407 = Unbundle By Name(w759) -> ("SRV"=w763:refnum<k5>)
        n408 = Variant To Data(error in=w768, type=FALSE ("Video Streaming"), Variant=w769) -> (data=w754:bool, error out=w760:errorcluster)
        n409 = case shown="True" w754 {
          tunnel: w763 -> [w774 w784]
          tunnel: [w774 w783] -> w762
          tunnel: w760 -> [w775 w779]
          tunnel: [w775 w782] -> w761
          tunnel: w759 -> [_ w776]
          frame False {
          }
          frame True {
            n410 = call "SRV_Main Config Paths.vi"("local data"=w776) -> ("SystemConfig Filepath"=w777:path)  [unwired: 8 in, 6 out]
            n411 = call "SRV_Read System Config File.vi"("System Config File Path"=w777, "error in (no error)"=w779) -> ("System Config"=w780:T29, "error out"=w778:errorcluster)  [unwired: 10 in, 2 out]
            n412 = Unbundle By Name(w780) -> ("Video Stream Rate Period (ms)"=w785:u32)
            n413 = call "SRV_Build Video Stream Rate Command.vi"("Video Stream Rate Period (ms)"=w785) -> ("Command String"=w781:string)  [unwired: 9 in, 1 out]
            n414 = call "SRV_Write_Comm.vi"("error in (no error)"=w778, "Command Sent"=w781, "SRV In"=w784) -> ("error out"=w782:errorcluster, "SRV Out"=w783:refnum<k5>)  [unwired: 6 in, 1 out]
          }
        }
        n415 = case shown="False" w754 {
          frame False {
            n416 = property on="Movie" class="Bool (strict)"("Val(Sgnl)"=FALSE ("Movie")) -> ()  [unwired: 2 in, 2 out]
          }
          frame True {
          }
        }
        n417 = Select(t=w766, s=w754, f=w765) -> (s? t:f=w758:string)
        n418 = Select(t=T20."Enabled" ("Disabled"), s=w754, f=T20."Disabled and Grayed Out" ("Disabled")) -> (s? t:f=w755:T20)
        n419 = property on="Camera" class="Bool"("DisabledEnum"=w755) -> ()  [unwired: 2 in, 2 out]
        n420 = property on="Movie" class="Bool (strict)"("DisabledEnum"=w755) -> ()  [unwired: 2 in, 2 out]
        n421 = call "SRV_Write_Comm.vi"("error in (no error)"=w761, "Command Sent"=w758, "SRV In"=w762) -> ("error out"=w772:errorcluster, "SRV Out"=w770:refnum<k5>)  [unwired: 6 in, 1 out]
        n422 = call "SRV_Update Streaming States VIG.vi"("Enabled"=w754, "Streaming Modes"=SRV_Streaming_Modes."Video") -> ()  [unwired: 14 in]
        n423 = Bundle By Name(cluster=w759, "SRV"=w770) -> (w771:T11)
      }
      frame "Clear" {
        n424 = Unbundle By Name(w787) -> ("Replies"=w786:refnum<vi>)
        n425 = call "SRV_Update Replies Indicator.vi"("Replies ref"=w786, "Text to Append"="xXxClearRepliesxXx", "error in (no error)"=w790) -> ("error out"=w789:errorcluster)  [unwired: 11 in, 1 out]
      }
      frame "Read PicoC Buffer" {
        n426 = Unbundle By Name(w791) -> ("SRV"=w794:refnum<k5>)
        n427 = call "SRV_Write_Comm.vi"("error in (no error)"=w796, "Command Sent"="*B\r", "SRV In"=w794) -> ("error out"=w795:errorcluster, "SRV Out"=w792:refnum<k5>)  [unwired: 6 in, 1 out]
        n428 = Bundle By Name(cluster=w791, "SRV"=w792) -> (w793:T11)
      }
      frame "CCode" {
        n429 = Unbundle By Name(w811) -> ("Replies"=w810:refnum<vi>, "SRV"=w801:refnum<k5>, "Status"=w809:refnum<vi>)
        n430 = call "SRV_Update Status Indicator.vi"("Status ref"=w809, "Status"="Waiting to load C Code...", "error in (no error)"=w819) -> ("Status ref out"=w818:refnum<vi>, "error out"=w820:errorcluster)  [unwired: 11 in]
        n431 = call "SRV_Wait for Zero IMJ Requests.vi"("Number of IMJ Requests ref"=w821, "#IMJ semaphore ref"=w816, "error in (no error)"=w820) -> ("error out"=w822:errorcluster)  [unwired: 10 in, 2 out]
        n432 = call <vilib>:"Acquire Semaphore.vi"("error in (no error)"=w822, "semaphore"=w830) -> ("error out"=w825:errorcluster, "semaphore out"=w828:T23)  [unwired: 3 in, 1 out]
        n433 = call "SRV_Update Status Indicator.vi"("Status ref"=w818, "Status"="Loading C Code...", "error in (no error)"=w825, "Delay After Update (0 ms)"=u32 500) -> ("Status ref out"=w824:refnum<vi>, "error out"=w806:errorcluster)  [unwired: 10 in]
        n434 = call "SRV_PM_App Initialization Routine.vi"("Packet Mode Enable (T)"=FALSE, "Read Response (F)"=TRUE, "error in (no error)"=w806, "connection ID"=w801) -> ("error out"=w805:errorcluster, "connection ID out"=w800:refnum<k5>)  [unwired: 4 in, 2 out]
        n435 = call "SRV_XModem_WriteFile_Comm.vi"("error in (no error)"=w805, "File Contents"="C Code", "SRV In"=w800) -> ("error out"=w804:errorcluster, "SRV Out"=w799:refnum<k5>, "## Reply"=w814:string, "Replies"=w823:string[])  [unwired: 4 in, 1 out]
        n436 = local write "XModem Replies"(w823) -> ()
        n437 = call "SRV_PM_App Initialization Routine.vi"("Packet Mode Enable (T)"=TRUE, "error in (no error)"=w804, "connection ID"=w799) -> ("error out"=w803:errorcluster, "connection ID out"=w798:refnum<k5>)  [unwired: 5 in, 2 out]
        n438 = call "SRV_Update Status Indicator.vi"("Status ref"=w824, "error in (no error)"=w803) -> ("error out"=w813:errorcluster)  [unwired: 12 in, 1 out]
        n439 = call "SRV_Update Replies Indicator.vi"("Replies ref"=w810, "Text to Append"=w814, "error in (no error)"=w813) -> ("error out"=w815:errorcluster)  [unwired: 11 in, 1 out]
        n440 = Bundle By Name(cluster=w811, "SRV"=w798) -> (w812:T11)
        n441 = call <vilib>:"Release Semaphore.vi"("error in (no error)"=w815, "semaphore"=w828) -> ("error out"=w829:errorcluster)  [unwired: 4 in, 1 out]
      }
      frame "Upload" {
        n442 = Unbundle By Name(w844) -> ("Replies"=w845:refnum<vi>, "SRV"=w839:refnum<k5>, "Status"=w843:refnum<vi>)
        n443 = call "SRV_Update Status Indicator.vi"("Status ref"=w843, "Status"="Waiting to load firmware...", "error in (no error)"=w854) -> ("Status ref out"=w853:refnum<vi>, "error out"=w855:errorcluster)  [unwired: 11 in]
        n444 = call "SRV_Wait for Zero IMJ Requests.vi"("Number of IMJ Requests ref"=w856, "#IMJ semaphore ref"=w850, "error in (no error)"=w855) -> ("error out"=w857:errorcluster)  [unwired: 10 in, 2 out]
        n445 = call <vilib>:"Acquire Semaphore.vi"("error in (no error)"=w857, "semaphore"=w867) -> ("error out"=w865:errorcluster, "semaphore out"=w866:T23)  [unwired: 3 in, 1 out]
        n446 = call "SRV_Update Status Indicator.vi"("Status ref"=w853, "Status"="Loading Firmware...", "error in (no error)"=w865, "Delay After Update (0 ms)"=u32 250) -> ("Status ref out"=w863:refnum<vi>, "error out"=w842:errorcluster)  [unwired: 10 in]
        n447 = call "SRV_PM_App Initialization Routine.vi"("Packet Mode Enable (T)"=FALSE, "Read Response (F)"=TRUE, "error in (no error)"=w842, "connection ID"=w839) -> ("error out"=w841:errorcluster, "connection ID out"=w840:refnum<k5>)  [unwired: 4 in, 2 out]
        n448 = Read from Binary File(8:w841, 10:-1 ("count (1)"), 11:"firmware") -> (0:w860:errorcluster, 2:w859:string)  [unwired: 3 in, 2 out]
        n449 = call "SRV_XModem_WriteFile_Comm.vi"("error in (no error)"=w860, "File Contents"=w859, "SRV In"=w840) -> ("error out"=w836:errorcluster, "SRV Out"=w833:refnum<k5>, "## Reply"=w848:string, "Replies"=→"XModem Replies":string[])  [unwired: 4 in, 1 out]
        n450 = call "SRV_PM_App Initialization Routine.vi"("Packet Mode Enable (T)"=TRUE, "error in (no error)"=w836, "connection ID"=w833) -> ("error out"=w835:errorcluster, "connection ID out"=w832:refnum<k5>)  [unwired: 5 in, 2 out]
        n451 = call "SRV_Update Status Indicator.vi"("Status ref"=w863, "error in (no error)"=w835) -> ("error out"=w847:errorcluster)  [unwired: 12 in, 1 out]
        n452 = call "SRV_Update Replies Indicator.vi"("Replies ref"=w845, "Text to Append"=w848, "error in (no error)"=w847) -> ("error out"=w849:errorcluster)  [unwired: 11 in, 1 out]
        n453 = Bundle By Name(cluster=w844, "SRV"=w832) -> (w846:T11)
        n454 = call <vilib>:"Release Semaphore.vi"("error in (no error)"=w849, "semaphore"=w866) -> ("error out"=w851:errorcluster)  [unwired: 4 in, 1 out]
      }
      frame "Boot" {
        # "Reboot the blackfin processor.\nThis will not disconnect the radio. It will emerge from the reboot not in packet mode, so read the reboot response on its own and then turn packet mode back on."
        # "copy the firmware from RAM into flash"
        # "Wait for response."
        n455 = Unbundle By Name(w904) -> ("Replies"=w892:refnum<vi>, "SRV"=w906:refnum<k5>, "Status"=w903:refnum<vi>)
        n456 = call "SRV_Update Status Indicator.vi"("Status ref"=w903, "Status"="Copying firmware from RAM into flash (zZ)...", "error in (no error)"=w911, "Delay After Update (0 ms)"=u32 100) -> ("Status ref out"=w908:refnum<vi>, "error out"=w869:errorcluster)  [unwired: 10 in]
        n457 = call "Log_TCP.vi"("Data"="zZ" ("data in"), "error in (no error)"=w869) -> ("Data dup"=w871:string, "error out"=w870:errorcluster)  [unwired: 12 in]
        n458 = call "SRV_Write_Comm.vi"("error in (no error)"=w870, "Command Sent"=w871, "SRV In"=w906) -> ("error out"=w902:errorcluster, "SRV Out"=w914:refnum<k5>)  [unwired: 6 in, 1 out]
        n459 = call "SRV_SRV_zZ Notifier.vi"("Notifier Methods"=SRV_SRV_Loops_Notifier_Methods."Wait on Notification", "error in (no error)"=w902, "timeout in ms (-1)"=10000) -> ("error out"=w897:errorcluster)  [unwired: 8 in]
        n460 = call "SRV_Update Status Indicator.vi"("Status ref"=w908, "Status"="Rebooting the processor ($!)...", "error in (no error)"=w897, "Delay After Update (0 ms)"=u32 250) -> ("Status ref out"=w907:refnum<vi>, "error out"=w896:errorcluster)  [unwired: 10 in]
        n461 = call <vilib>:"Acquire Semaphore.vi"("error in (no error)"=w896, "semaphore"=w893) -> ("error out"=w880:errorcluster, "semaphore out"=w894:T23)  [unwired: 3 in, 1 out]
        n462 = call "Log_TCP.vi"("Data"="$!" ("data in"), "error in (no error)"=w880) -> ("Data dup"=w878:string, "error out"=w881:errorcluster)  [unwired: 12 in]
        n463 = call "SRV_Write_Comm.vi"("error in (no error)"=w881, "Command Sent"=w878, "SRV In"=w914) -> ("error out"=w889:errorcluster, "SRV Out"=w890:refnum<k5>)  [unwired: 6 in, 1 out]
        n464 = call "SRV_Read_Comm_Response after Reboot.vi"("error in (no error)"=w889, "SRV In"=w890) -> ("error out"=w877:errorcluster, "Data out"=w874:string, "SRV Out"=w885:refnum<k5>)  [unwired: 7 in]
        n465 = call "Log_TCP.vi"("Data"=w874, "error in (no error)"=w877, "Response? (F: LV Writes)"=TRUE) -> ("Data dup"=w873:string, "error out"=w876:errorcluster)  [unwired: 11 in]
        n466 = call "SRV_Update Replies Indicator.vi"("Replies ref"=w892, "Text to Append"=w873, "error in (no error)"=w876) -> ("Replies ref out"=w884:refnum<vi>, "error out"=w886:errorcluster)  [unwired: 11 in]
        n467 = call "SRV_PM_App Initialization Routine.vi"("Packet Mode Enable (T)"=TRUE, "Read Response (F)"=TRUE, "error in (no error)"=w886, "connection ID"=w885) -> ("error out"=w883:errorcluster, "connection ID out"=w898:refnum<k5>, "Response"=w882:string)  [unwired: 4 in, 1 out]
        n468 = call "SRV_Update Replies Indicator.vi"("Replies ref"=w884, "Text to Append"=w882, "error in (no error)"=w883) -> ("error out"=w891:errorcluster)  [unwired: 11 in, 1 out]
        n469 = call <vilib>:"Release Semaphore.vi"("error in (no error)"=w891, "semaphore"=w894) -> ("error out"=w895:errorcluster)  [unwired: 4 in, 1 out]
        n470 = Bundle By Name(cluster=w904, "SRV"=w898) -> (w905:T11)
        n471 = call "SRV_Update Status Indicator.vi"("Status ref"=w907, "error in (no error)"=w895) -> ("error out"=w899:errorcluster)  [unwired: 12 in, 1 out]
      }
      frame "EdgHorzObj Detection" {
        n472 = Unbundle By Name(w920) -> ("SRV"=w922:refnum<k5>)
        n473 = call "CameraSetup.vi"("error in (no error)"=w923, "Task"=T25."Disable", "SRV In"=w922) -> ("error out"=w924:errorcluster, "SRV Out"=w925:refnum<k5>)  [unwired: 7 in]
        n474 = To Unsigned Word Integer(number="Plan") -> (unsigned 16bit integer=w927:u16)
        n475 = call "CameraSetup.vi"("error in (no error)"=w924, "Task"=w927, "SRV In"=w925) -> ("error out"=w915:errorcluster, "SRV Out"=w918:refnum<k5>)  [unwired: 7 in]
        n476 = call "Camera_EdgHorzObjThreshold.vi"("error in (no error)"=w915, "Threshold"="Threshold", "SRV In"=w918) -> ("error out"=w916:errorcluster, "SRV Out"=w917:refnum<k5>)  [unwired: 7 in]
        n477 = Bundle By Name(cluster=w920, "SRV"=w917) -> (w921:T11)
      }
      frame "QR Code Detection" {
        n478 = Unbundle By Name(w937) -> ("SRV"=w935:refnum<k5>)
        n479 = Variant To Data(error in=w933, type=QR_Code_Detection_Radio_Buttons."Nothing" ("QR Code Detection"), Variant=w931) -> (data=w929:T5, error out=w932:errorcluster)
        n480 = call "Camera_QR Code Detection.vi"("error in (no error)"=w932, "QR Code Detection"=w929, "SRV In"=w935) -> ("error out"=w936:errorcluster, "SRV Out"=w934:refnum<k5>)  [unwired: 7 in]
        n481 = Bundle By Name(cluster=w937, "SRV"=w934) -> (w938:T11)
      }
      frame "Color Segmentation" {
        n482 = Unbundle By Name(w946) -> ("SRV"=w948:refnum<k5>)
        n483 = call "CameraSetup.vi"("error in (no error)"=w949, "Task"=T25."Disable", "SRV In"=w948) -> ("error out"=w950:errorcluster, "SRV Out"=w951:refnum<k5>)  [unwired: 7 in]
        n484 = To Unsigned Word Integer(number="Plan 2") -> (unsigned 16bit integer=w953:u16)
        n485 = call "CameraSetup.vi"("error in (no error)"=w950, "Task"=w953, "SRV In"=w951) -> ("error out"=w940:errorcluster, "SRV Out"=w942:refnum<k5>)  [unwired: 7 in]
        n486 = To Unsigned Word Integer(number="vz Bins") -> (unsigned 16bit integer=w943:u16)
        n487 = call "Camera_ColorSegmentation.vi"("error in (no error)"=w940, "Bins"=w943, "SRV In"=w942) -> ("error out"=w939:errorcluster, "SRV Out"=w941:refnum<k5>)  [unwired: 7 in]
        n488 = Bundle By Name(cluster=w946, "SRV"=w941) -> (w947:T11)
      }
      frame "Motion Detection_Differencing" {
        n489 = Unbundle By Name(w955) -> ("SRV"=w958:refnum<k5>)
        n490 = call "CameraSetup.vi"("error in (no error)"=w960, "Task"=T25."Disable", "SRV In"=w958) -> ("error out"=w961:errorcluster, "SRV Out"=w962:refnum<k5>)  [unwired: 7 in]
        n491 = To Unsigned Word Integer(number="Plan 3") -> (unsigned 16bit integer=w964:u16)
        n492 = call "CameraSetup.vi"("error in (no error)"=w961, "Task"=w964, "SRV In"=w962) -> ("error out"=w959:errorcluster, "SRV Out"=w956:refnum<k5>)  [unwired: 7 in]
        n493 = Bundle By Name(cluster=w955, "SRV"=w956) -> (w957:T11)
      }
      frame "Motion Detection_Blobs" {
        n494 = Unbundle By Name(w968) -> ("SRV"=w970:refnum<k5>)
        n495 = call "CameraSetup.vi"("error in (no error)"=w971, "Task"=T25."Disable", "SRV In"=w970) -> ("error out"=w972:errorcluster, "SRV Out"=w973:refnum<k5>)  [unwired: 7 in]
        n496 = To Unsigned Word Integer(number="Plan 4") -> (unsigned 16bit integer=w975:u16)
        n497 = call "CameraSetup.vi"("error in (no error)"=w972, "Task"=w975, "SRV In"=w973) -> ("error out"=w965:errorcluster, "SRV Out"=w966:refnum<k5>)  [unwired: 7 in]
        n498 = Bundle By Name(cluster=w968, "SRV"=w966) -> (w969:T11)
      }
      frame "Blob Det_vc Bins" {
        n499 = Unbundle By Name(w976) -> ("SRV"=w979:refnum<k5>)
        n500 = To Unsigned Word Integer(number="vc Bins") -> (unsigned 16bit integer=w982:u16)
        n501 = call "Camera_BlobColorBin.vi"("error in (no error)"=w981, "Bins"=w982, "SRV In"=w979) -> ("error out"=w980:errorcluster, "SRV Out"=w977:refnum<k5>)  [unwired: 7 in]
        n502 = Bundle By Name(cluster=w976, "SRV"=w977) -> (w978:T11)
      }
      frame "Camera" {
        n503 = call "SRV_Check-Establish Directory Path.vi"("error in (no error)"=w987, "Directory Path"="Images Directory Path") -> ("error out"=w986:errorcluster, "Directory Path dup"=w984:path)  [unwired: 8 in]
        n504 = call "SRV_VIG_Camera.vi"("Camera"=TRUE, "Images Directory Path"=w984, "Method (Get)"=enum16{"Get", "Set"}."Set") -> ()  [unwired: 11 in, 2 out]
      }
      frame "Movie" {
        n505 = Variant To Data(error in=w996, type=FALSE ("Movie"), Variant=w997) -> (data=w992:bool, error out=w994:errorcluster)
        n506 = case shown="True" w992 {
          tunnel: [_ w1006] -> w995
          tunnel: w994 -> [w1001 w1005]
          tunnel: [w1001 w1004] -> w993
          tunnel: [enum16{"Get", "Start", "Stop"}."Stop" ("Method (Get)") enum16{"Get", "Start", "Stop"}."Start" ("Method (Get)")] -> w991
          frame False {
          }
          frame True {
            n507 = local read "Images Directory Path"() -> (w1002:path)
            n508 = call "SRV_Check-Establish Directory Path.vi"("error in (no error)"=w1005, "Directory Path"=w1002) -> ("error out"=w1004:errorcluster, "Directory Path dup"=w1006:path)  [unwired: 8 in]
          }
        }
        n509 = call "SRV_VIG_Movie.vi"("Images Directory Path"=w995, "Method (Get)"=w991) -> ()  [unwired: 10 in, 4 out]
      }
      frame "RGB" {
        w1007 = T31 {"Witdh"=0, "Height"=0, "Depth"=0, "data"=[], "Compressed data"=[], "Color table"=[], "Duration"=0, "Options"=0, "Timestamp"=0, "ID"=0, "Reserved"=0, "Dialogs"=0}  # Image/Movie Out
        # "was an old indicator on the front panel that has long been unused.\nOnce upon a time, it had been updated with the ##IMJ data."
        n510 = property on="The image" class="Pict"(error in=w1013) -> (error out=w1014:errorcluster, "Mouse"=w1018:T32)  [unwired: 1 in, 1 out]
        n511 = Unbundle By Name(w1018) -> ("Mouse Position"=w1017:cluster{"X":i32, "Y":i32})
        n512 = Unbundle By Name(w1008) -> ("SRV"=w1011:refnum<k5>)
        n513 = Unbundle(w1017) -> ("X"=w1016:i32, "Y"=w1015:i32)
        n514 = call "LV86_Get Pixel Value.vi"("Position"=w1017, "Image In"=w1007) -> ("RGB"=w1025:cluster{"R":u32, "G":u32, "B":u32})  [unwired: 1 in, 2 out]
        n515 = Divide(x=w1025, y=255) -> (x/y=w1022:cluster{"R":dbl, "G":dbl, "B":dbl})
        n516 = Format Into String(format string="vp%04d%04d", error in=w1014, w1016, w1015) -> (resulting string=w1020:string, error out=w1019:errorcluster)  [unwired: 1 in]
        n517 = call "RGB-HSV.vi"("RGB"=w1022) -> ("YUV"=→"YUV_Calc":cluster{"Y":sgl, "U":sgl, "V":sgl})  [unwired: 13 in, 1 out]
        n518 = call "SRV_Write_Comm.vi"("error in (no error)"=w1019, "Command Sent"=w1020, "SRV In"=w1011) -> ("error out"=w1012:errorcluster, "SRV Out"=w1009:refnum<k5>)  [unwired: 6 in, 1 out]
        n519 = Bundle By Name(cluster=w1008, "SRV"=w1009) -> (w1010:T11)
      }
      frame "Edit System Config" {
        n520 = call "SRV_Main Config Paths.vi"("local data"=w1027) -> ("SystemConfig Filepath"=w1026:path)  [unwired: 8 in, 6 out]
        n521 = call "SRV_System Config GUI.vi"("System Config File Path in"=w1026) -> ("error out"=w1032:errorcluster, "Cancelled?"=w1028:bool)  [unwired: 8 in, 1 out]
        n522 = Select(t=w1033, s=w1033, f=w1032) -> (s? t:f=w1031:errorcluster)
        n523 = case "Cancelled?" shown="False" w1028 {
          tunnel: w1031 -> [w1037 w1038]
          tunnel: [w1036 w1038] -> w1030
          tunnel: w1029 -> [w1035 _]
          frame False {
            n524 = call "SRV_Queue_Enqueue Element.vi"("error in (no error)"=w1037, "Command"="InitTCP", "Command-Data Queue"=w1035) -> ("error out"=w1036:errorcluster)  [unwired: 6 in, 2 out]
          }
          frame True {
          }
        }
      }
      frame "Edit Motors Config" {
        n525 = call "SRV_Main Config Paths.vi"("local data"=w1040) -> ("MotorsConfig Filepath"=w1039:path)  [unwired: 8 in, 6 out]
        n526 = call "SRV_Motors Config GUI.vi"("Motors Config File Path in"=w1039) -> ("error out"=w1045:errorcluster, "Cancelled?"=w1041:bool)  [unwired: 8 in, 1 out]
        n527 = Select(t=w1046, s=w1046, f=w1045) -> (s? t:f=w1044:errorcluster)
        n528 = case "Cancelled?" shown="False" w1041 {
          tunnel: w1044 -> [w1050 w1051]
          tunnel: [w1049 w1051] -> w1043
          tunnel: w1042 -> [w1048 _]
          frame False {
            n529 = call "SRV_Queue_Enqueue Element.vi"("error in (no error)"=w1050, "Command"="InitMotors", "Command-Data Queue"=w1048) -> ("error out"=w1049:errorcluster)  [unwired: 6 in, 2 out]
          }
          frame True {
          }
        }
      }
      frame "Edit Sensors Config" {
        n530 = call "SRV_Main Config Paths.vi"("local data"=w1053) -> ("SensorsConfig Filepath"=w1052:path)  [unwired: 8 in, 6 out]
        n531 = call "SRV_Sensors Config GUI.vi"("Sensors Config File Path in"=w1052) -> ("error out"=w1058:errorcluster, "Cancelled?"=w1054:bool)  [unwired: 8 in, 1 out]
        n532 = Select(t=w1059, s=w1059, f=w1058) -> (s? t:f=w1057:errorcluster)
        n533 = case "Cancelled?" shown="False" w1054 {
          tunnel: w1057 -> [w1061 w1067]
          tunnel: [w1060 w1067] -> w1056
          tunnel: w1055 -> [_ _]
          frame False {
            n534 = call "SRV_VIG_Sensor View Tab Open.vi"() -> ("Sensor View Tab Open?"=w1062:bool)  [unwired: 14 in, 1 out]
            n535 = case "Sensor View Tab Open?" shown="True" w1062 {
              tunnel: w1061 -> [w1063 w1066]
              tunnel: [w1063 w1065] -> w1060
              frame False {
              }
              frame True {
                n536 = call "SRV_SensorsQueue_Enqueue Element.vi"("error in (no error)"=w1066, "Command"="Initialize") -> ("error out"=w1065:errorcluster)  [unwired: 9 in]
              }
            }
          }
          frame True {
          }
        }
      }
      frame "Button Value Change" {
        n537 = Unbundle By Name(w1086) -> ("SRV"=w1083:refnum<k5>, "true refs"=w1079:refnum<vi>[], "Motor Control Config"=w1072:T12[])
        n538 = Variant To Data(error in=w1080, type=T24 {"Button NewVal"=FALSE, "Button Index"=-1} ("Button Event Data"), Variant=w1081) -> (data=w1076:T24, error out=w1075:errorcluster)
        n539 = Unbundle By Name(w1076) -> ("Button Index"=w1073:i32, "Button NewVal"=w1071:bool)
        n540 = Index Array(array=w1079, index=w1073) -> (element=w1078:refnum<vi>)
        n541 = Index Array(array=w1072, index=w1073) -> (element=w1069:T12)
        n542 = case shown="True" w1071 {
          tunnel: w1069 -> [w1088 w1090]
          tunnel: [w1087 w1089] -> w1070
          frame True {
            n543 = Unbundle By Name(w1088) -> ("Press Cmds.Motor Control Commands Array"=w1087:T15[])
          }
          frame False {
            n544 = Unbundle By Name(w1090) -> ("Release Cmds.Motor Control Commands Array"=w1089:T15[])
          }
        }
        n545 = property class="Ring (strict)"(reference=w1078, error in=w1075, "Visible"=w1071) -> (error out=w1074:errorcluster)  [unwired: 1 out]
        n546 = Unbundle By Name(w1069) -> ("Motor Type"=w1068:T13)
        n547 = call "SRV_Execute Multiple Motor Control Commands.vi"("SRV"=w1083, "Motor Type"=w1068, "Motor Control Commands"=w1070, "error in (no error)"=w1074) -> ("SRV Out"=w1084:refnum<k5>, "error out"=w1082:errorcluster)  [unwired: 9 in, 1 out]
        n548 = Bundle By Name(cluster=w1086, "SRV"=w1084) -> (w1085:T11)
      }
      frame "Close Sensor View" {
        n549 = call "SRV_SensorsQueue_Enqueue Element.vi"("Ignore Error 1? (F)"=TRUE, "error in (no error)"=w1096, "Command"="Exit") -> ("error out"=w1094:errorcluster)  [unwired: 8 in]
        n550 = flat-sequence {
          tunnel: w1094 -> [w1099]
          tunnel: [w1099] -> w1093
          frame #0 {
            n551 = call "SRV_Update Streaming States VIG.vi"("Enabled"=FALSE, "Streaming Modes"=SRV_Streaming_Modes."Sensors") -> ()  [unwired: 14 in]
          }
        }
        n552 = call "SRV_Wait (ms)+.vi"("milliseconds to wait"=u32 100, "error in (no error)"=w1093) -> ("error out"=w1092:errorcluster)  [unwired: 12 in, 1 out]
      }
      frame "Cache Streaming States" {
        n553 = call "SRV_VIG_XModem Updates in Progress.vi"("XModem Updates in Progress"=TRUE, "Method (Get)"=enum16{"Get", "Set"}."Set") -> ()  [unwired: 12 in, 2 out]
        n554 = call "SRV_VIG_Streaming States.vi"() -> ("Streaming States out"=w1104:T16)  [unwired: 15 in]
        n555 = Bundle By Name(cluster=w1106, "Cached Streaming States"=w1104) -> (w1105:T11)
      }
      frame "Restore Streaming States" {
        n556 = Unbundle By Name(w1116) -> ("Cached Streaming States"=w1115:T16)
        n557 = call "SRV_Queue Streaming Restore States.vi"("error in (no error)"=w1113, "Cached Streaming States"=w1115, "Control Queue"=w1114) -> ("error out"=w1111:errorcluster)  [unwired: 7 in, 1 out]
        n558 = call "SRV_VIG_XModem Updates in Progress.vi"("XModem Updates in Progress"=FALSE, "Method (Get)"=enum16{"Get", "Set"}."Set") -> ()  [unwired: 12 in, 2 out]
        n559 = property on="Show Image" class="Bool (strict)"(error in=w1111, "DisabledEnum"=T20."Enabled" ("Disabled")) -> (error out=w1110:errorcluster)  [unwired: 1 in, 1 out]
      }
      frame "Developer Error", Default {
        n560 = Format Into String(format string="Developer Error: The command \"%s\" is undefined for the Control Queue.", w1120) -> (resulting string=w1118:string)  [unwired: 2 in, 1 out]
        n561 = call "SRV_Generate Error.vi"("Message"=w1118, "error in (no error)"=w1117) -> ("error out"=w1119:errorcluster)  [unwired: 13 in]
      }
      frame "CloseTCP" {
        n562 = Unbundle By Name(w1123) -> ("SRV"=w1126:refnum<k5>)
        n563 = call "SRV_Close TCP Connection.vi"("error in"=w1128, "connection ID"=w1126) -> ("error out"=w1127:errorcluster)  [unwired: 9 in]
        n564 = Bundle By Name(cluster=w1123, "SRV"=refnum<k5> refnum ("SRV Out")) -> (w1125:T11)
      }
      frame "Done" {
        n565 = Unbundle By Name(w1144) -> ("button refs"=w1131:refnum<vi>[], "false refs"=w1130:refnum<vi>[], "true refs"=w1129:refnum<vi>[], "Status"=w1143:refnum<vi>)
        n566 = global read "SRVGlobals.vi" "Connected SRV IP"() -> (w1154:string[])
        n567 = call "SRV_Update Status Indicator.vi"("Status ref"=w1143, "Status"="Exiting...", "error in (no error)"=w1152) -> ("error out"=w1142:errorcluster)  [unwired: 11 in, 1 out]
        n568 = Release Queue(queue=w1140, error in (no error)=w1142) -> (error out=w1141:errorcluster)  [unwired: 1 in, 2 out]
        n569 = for {
          tunnel: w1154 -> [w1165] mode=indexing
          shift-right: [w1162] -> _
          shift-left: errorcluster {"status"=FALSE, "code"=0, "source"=""} ("error out") -> [w1163]
          n570 = call "SRV_Reset TCP Connection.vi"("IP address"=w1165) -> ("error out"=w1164:errorcluster)  [unwired: 9 in, 1 out]
          n571 = Select(t=w1163, s=w1163, f=w1164) -> (s? t:f=w1162:errorcluster)
        }
        n572 = Release Queue(queue=w1145, error in (no error)=w1141) -> (error out=w1146:errorcluster)  [unwired: 1 in, 2 out]
        n573 = call "SRV_Number of IMJ Requests Methods.vi"("Number of IMJ Requests ref"=w1147, "semaphore ref"=w1148, "error in (no error)"=w1146, "Number of IMJ Requests Methods (Read)"=SRV_Number_of_IMJ_Requests_Methods."Close") -> ("error out"=w1133:errorcluster)  [unwired: 7 in, 4 out]
        n574 = disable-structure shown="Disabled" {
          disable-tunnel: w1133 -> [w1160 w1161]
          disable-tunnel: [w1159 w1161] -> w1132
          disable-tunnel: w1131 -> [w1158 _]
          disable-tunnel: w1130 -> [w1157 _]
          disable-tunnel: w1129 -> [w1156 _]
          frame Disabled {
            n575 = call "SRV_Shutdown Motor Buttons.vi"("button refs"=w1158, "false refs"=w1157, "true refs"=w1156, "error in (no error)"=w1160) -> ("error out"=w1159:errorcluster)  [unwired: 11 in]
          }
          frame Enabled {
          }
        }
        n576 = call "SRV_SRV_Loops Notifier.vi"("Notifier Methods"=SRV_SRV_Loops_Notifier_Methods."Release Notifier", "error in (no error)"=w1132) -> ("error out"=w1139:errorcluster)  [unwired: 8 in, 1 out]
        n577 = call "SRV_SRV_zZ Notifier.vi"("Notifier Methods"=SRV_SRV_Loops_Notifier_Methods."Release Notifier", "error in (no error)"=w1139) -> ("error out"=w1137:errorcluster)  [unwired: 9 in]
        n578 = call "SRV_SensorsQueue_Enqueue Element.vi"("Ignore Error 1? (F)"=TRUE, "error in (no error)"=w1137, "Command"="Exit") -> ("error out"=w1136:errorcluster)  [unwired: 8 in]
      }
    }
    n579 = Unbundle By Name(w430) -> ("SRV"=w429:refnum<k5>)
    n580 = Not A Number/Path/Refnum?(number/path/refnum=w429) -> (NaN/Path/Refnum?=w444:bool)
    n581 = Not(x=w444) -> (.not. x?=→"connected?":bool)
    n582 = call "SRV_Manage Loop Errors.vi"("Loop Identifier"="Control Loop", "error in (no error)"=w426) -> ("error out"=w432:errorcluster)  [unwired: 9 in]
    "i2" <- w437
  }
  n583 = while {
    tunnel: w111 -> [w1202]
    tunnel: [w1199] -> w117
    tunnel: w140 -> [w1197]
    shift-right: [w1190] -> _
    shift-left: w113 -> [w1180]
    tunnel: w2 -> [w1194]
    tunnel: w141 -> [w1193]
    tunnel: w138 -> [w1187]
    tunnel: w116 -> [w1181]
    tunnel: w112 -> [w1166]
    i -> [w1198]
    stop <- w1203 stop-if-true
    # "# IMJ Requests sema"
    # "# IMJ Requests ref"
    # "SRV IP"
    n584 = call "SRV_ms Timer.vi"("error in (no error)"=w1180) -> ("ms Tick"=w1174:u32, "error out"=w1179:errorcluster)  [unwired: 16 in, 1 out]
    n585 = call "SRV_PM_Dequeue and Parse Packet.vi"("SRV_Packets queue"=w1181, "error in (no error)"=w1179) -> ("Packet"=w1189:T19, "Data String"=w1188:string, "error out"=w1176:errorcluster)  [unwired: 4 in, 7 out]
    n586 = case shown="\"New PM\"" w1187 {
      tunnel: w1202 -> [w1213 w1214]
      tunnel: [w1212 w1214] -> w1201
      frame "Old" {
        n587 = call <vilib>:"Acquire Semaphore.vi"("semaphore"=w1213) -> ("semaphore out"=w1212:T23)  [unwired: 4 in, 2 out]
      }
      frame "New PM" {
        # "TCP Read sema"
      }
    }
    n588 = call "SRV_PM_VIG_WIP Byte Array Size.vi"() -> ("WIP Size out"=w1170:i32)  [unwired: 10 in, 1 out]
    n589 = call "SRV_ms Timer.vi"("ms Previous Tick"=w1174, "error in (no error)"=w1176) -> ("ms Tick"=w1173:u32, "ms Diff"=→"ms Diff DQ":u32, "error out"=w1175:errorcluster)  [unwired: 15 in]
    n590 = call "SRV_Determine Incoming Data Type.vi"("Data"=w1188, "error in (no error)"=w1175) -> ("Data dup"=w1186:string, "Response Data Type"=w1183:T3, "error out"=w1184:errorcluster)  [unwired: 11 in]
    n591 = Greater?(x=w1170, y=100000) -> (0:→"Overflow Indicator":bool)
    n592 = call "SRV_Send No Data if Shutdown.vi"("Data"=w1186, "Response Data Type"=w1183, "error in (no error)"=w1184) -> ("Data dup"=w1185:string, "Response Data Type out"=w1182:T3, "error out"=w1178:errorcluster)  [unwired: 10 in]
    "Response Data Type" <- w1182
    n593 = call "SRV_ms Timer.vi"("ms Previous Tick"=w1173, "error in (no error)"=w1178) -> ("ms Diff"=→"ms Diff parse":u32, "error out"=w1177:errorcluster)  [unwired: 15 in, 1 out]
    n594 = case shown="\"##IMJ\"" w1182 {
      selector: w1182 -> [_ _ _ _ _ _ _ w1296 _]
      tunnel: w1166 -> [_ w1231 _ _ _ _ _ _ _]
      tunnel: [w1216 _ w1263 w1269 w1274 w1284 w1289 _ w1316] -> w1196
      tunnel: [_ _ _ _ _ _ _ _ w1307] -> w1203
      tunnel: w1201 -> [w1221 w1232 w1265 w1271 w1282 w1287 w1294 w1300 w1317]
      tunnel: [w1221 w1232 w1265 w1271 w1282 w1287 w1294 w1300 w1317] -> w1200
      tunnel: w1197 -> [_ w1229 _ _ _ _ _ _ _]
      tunnel: [w1219 w1224 w1258 w1270 w1272 w1285 w1291 w1298 w1308] -> w1195
      tunnel: w1177 -> [w1220 w1227 w1259 w1270 w1273 w1286 w1292 w1299 w1309]
      tunnel: w1193 -> [_ w1228 _ _ _ _ _ _ _]
      tunnel: w1189 -> [_ _ _ _ _ _ _ _ _]
      tunnel: w1185 -> [w1217 w1230 w1264 w1269 w1274 w1284 w1289 w1297 w1316]
      frame "Undefined Data" {
        n595 = call "SRV_Shutdown Flag.vi"("error in (no error)"=w1220) -> ("Shutdown Flag out"=w1218:bool, "error out"=w1219:errorcluster)  [unwired: 13 in]
        n596 = Select(t="", s=w1218, f=w1217) -> (s? t:f=w1216:string)
      }
      frame "##IMJ" {
        n597 = call "SRV_ms Timer.vi"("error in (no error)"=w1227) -> ("ms Tick"=w1223:u32, "error out"=w1226:errorcluster)  [unwired: 16 in, 1 out]
        n598 = flat-sequence {
          tunnel: w1231 -> [w1250]
          tunnel: w1226 -> [w1243]
          tunnel: [w1233] -> w1225
          tunnel: w1230 -> [w1248]
          tunnel: w1229 -> [_]
          tunnel: w1228 -> [_]
          frame #0 {
            # "TCP Reads if using old non-packet mode"
            # "grab JPEG compressed video frame"
            n599 = call "SRV_ms Timer.vi"("error in (no error)"=w1243) -> ("ms Tick"=w1239:u32, "error out"=w1242:errorcluster)  [unwired: 16 in, 1 out]
            n600 = call "SRV_Get TCP Connection.vi"("error in (no error)"=w1242, "IP address"=w1250) -> ("error out"=w1241:errorcluster, "connection ID"=w1249:refnum<k5>)  [unwired: 8 in]
            n601 = call "SRV_ms Timer.vi"("ms Previous Tick"=w1239, "error in (no error)"=w1241) -> ("ms Tick"=w1247:u32, "ms Diff"=→"ms Diff 2":u32, "error out"=w1244:errorcluster)  [unwired: 15 in]
            n602 = call "SRV_Get and Show Image.vi"("Connection ID"=w1249, "Data"=w1248, "error in (no error)"=w1244) -> ("image"=w1251:picture, "dimensions"=w1252:cluster{"Witdh":i32, "Height":i32}, "error out"=w1245:errorcluster)  [unwired: 8 in, 2 out]
            n603 = call "SRV_ms Timer.vi"("ms Previous Tick"=w1247, "error in (no error)"=w1245) -> ("ms Tick"=w1240:u32, "ms Diff"=→"ms Diff":u32, "error out"=w1237:errorcluster)  [unwired: 15 in]
            n604 = flat-sequence {
              tunnel: w1252 -> [w1257]
              tunnel: w1251 -> [w1253]
              tunnel: [w1254] -> w1234
              tunnel: w1240 -> [w1255]
              tunnel: w1237 -> [w1256]
              tunnel: [w1255] -> w1236
              frame #0 {
                n605 = property on="The image" class="Pict"("Draw Area Size"=w1257) -> ()  [unwired: 2 in, 2 out]
                n606 = call <vilib>:"Clear Errors.vi"("error in (no error)"=w1256) -> ("error out"=w1254:errorcluster)  [unwired: 5 in, 1 out]
                "The image" <- w1253
              }
            }
            n607 = call "SRV_ms Timer.vi"("ms Previous Tick"=w1236, "error in (no error)"=w1234) -> ("ms Diff"=→"ms Diff 3":u32, "error out"=w1233:errorcluster)  [unwired: 15 in, 1 out]
          }
        }
        n608 = call "SRV_ms Timer.vi"("ms Previous Tick"=w1223, "error in (no error)"=w1225) -> ("ms Diff"=→"ms Diff ##IMJ":u32, "error out"=w1224:errorcluster)  [unwired: 15 in, 1 out]
      }
      frame "#B" {
        # "Read the contents of the PicoC printf() buffer and clear it.\n\nThis command causes the contents of the PicoC buffered serial stream (from printf() and output() calls in PicoC, when the buffered mode is enabled) to be send in the reply. Note that the reply can be up to 64KB long. After the entire contents of the buffer are sent in the reply, the buffer is cleared.\n\n[length] is an ASCII value from 0 to 65525 and it indicates the number of bytes in [buffer_data].\n\n[buffer_data] is the entire contents of the serial stream buffer, and can include any data bytes"
        n609 = call "SRV_Parse Response (B).vi"("#B Data in"=w1264) -> ("number of bytes in buffer_data"=w1262:i32, "Beginning of buffer_data"=w1261:string)  [unwired: 4 in, 5 out]
        n610 = call "Log_B.vi"("Data"=w1261, "number of bytes in buffer_data"=w1262, "error in (no error)"=w1259) -> ("Data dup"=w1260:string, "error out"=w1258:errorcluster)  [unwired: 11 in]
        n611 = case shown="..0" w1262 {
          tunnel: w1260 -> [_ w1267]
          tunnel: ["" w1267] -> w1263
          frame ..0 {
          }
          frame 1.. {
          }
        }
      }
      frame "Leaving PicoC" {
        # "Execute C Program\n\nRuns the PicoC program stored in flash buffer, which got there via the 'E' line editor, the 'zr' or 'zRxx' command (which reads a flash sector into flash buffer) or 'X' command (XMODEM file transfer). PicoC program must have an exit(1); call to return control to the main firmware.\n\nWhen PicoC Background Mode mode is active (simultainous PicoC and Firmware commands), you must send a '|' character to get PicoC to exit before the exit(); call in the code. When PicoC Background Mode is not active (only PicoC running, Firmware commands ignored), you have to send an 'ESC' to terminate the PicoC program before the exit(); call runs.\n\nWhen PicoC exits, the SRV will send the string \"##Leaving PicoC\\r\\n\", which indicates to the client that the PicoC program exited normally.\n \n'|'  Break out of running PicoC program\n\nIf a PicoC program is running and PicoC Background Mode is active, you can send the '|' character to the firmware and at the next statement, the PicoC program will exit and return \"##Leaving PicoC\\r\\n\"."
        n612 = local write "In Pico"(FALSE ("Enable?")) -> ()
      }
      frame "##vp" {
        # "RGB\n\n##vp yyy uuu vvv\\r\\n\n\nthe 'vp' command samples a single pixel defined by coordinates xxxx (column 0000-0159, 0000-0319, 0000-0639, 0000-1279 depending on resolution) and yy (row 0000-0127, 0000-0255, 0000-0511, 0000-1023, where 0000 is top of image). 'vp01600128' will sample a pixel in the middle of the image at 320x256 resolution, 'vp01600000' will sample a pixel in the middle of the top row, etc..."
        n613 = Match Pattern(string=w1274, regular expression="vp " ("Command Sent")) -> (after substring=w1275:string)  [unwired: 1 in, 3 out]
        n614 = Scan From String(input string=w1275, error in=w1273) -> (error out=w1281:errorcluster, output 1=w1279:dbl, output 2=w1278:dbl, output 3=w1277:dbl)  [unwired: 5 in, 2 out]
        n615 = Bundle(w1279, w1278, w1277) -> (→"YUV_SRV":cluster{dbl, dbl, dbl})  [unwired: 1 in]
        n616 = call <vilib>:"Clear Errors.vi"("error in (no error)"=w1281) -> ("error out"=w1272:errorcluster)  [unwired: 5 in, 1 out]
      }
      frame "##zZ" {
        # "##zZ\\r\\n\n\nflash memory boot sector update - writes contents of flash buffer to boot sectors of flash memory - used to replace u-boot.ldr or srv1.ldr - checks first that a valid LDR format image is in the flash buffer"
        n617 = call "SRV_SRV_zZ Notifier.vi"("Notifier Methods"=SRV_SRV_Loops_Notifier_Methods."Send Notification", "error in (no error)"=w1286, "Notification String"=w1284) -> ("error out"=w1285:errorcluster)  [unwired: 8 in]
      }
      frame "##g:7" {
        # "##g:7\n\nIf, and only if, a valid QR tag is seen and decoded, the BFin will send a \"##g:7\" packet. (those will be the first 5 bytes of the payload). After those bytes, there will be a space, a single quote, then the value decoded from the QR tag, and then another single quote.\nThis ##g:7 packet will be sent immediately before the frame that contains the image where the QR code was recognized. So MasterControl can use the presence of this packet to set a flag so that the next image that comes in can be saved to a file."
        n618 = local read "Images Directory Path"() -> (w1288:path)
        n619 = call "SRV_Parse Response (QR Code).vi"("data"=w1289, "error in (no error)"=w1292) -> ("QR Code"=w1290:string, "error out"=w1291:errorcluster)  [unwired: 12 in]
        n620 = call "SRV_VIG_QR.vi"("QR Code"=w1290, "Images Directory Path"=w1288, "Method (Get and Reset)"=enum16{"Get and Reset", "Set"}."Set") -> ()  [unwired: 9 in, 4 out]
      }
      frame "##N$B".."##&R," {
        # "##N$B\n##N$b\n##i$l\n##i$L\n##i$N\n##&NP,\n##&R,"
        n621 = call "SRV_VIG_Sensor View Tab Open.vi"() -> ("Sensor View Tab Open?"=w1295:bool)  [unwired: 14 in, 1 out]
        n622 = case "Sensor View Tab Open?" shown="True" w1295 {
          tunnel: w1299 -> [w1301 w1306]
          tunnel: [w1301 w1305] -> w1298
          tunnel: w1297 -> [_ w1304]
          tunnel: w1296 -> [_ w1302]
          frame False {
          }
          frame True {
            n623 = Format Into String(w1302) -> (resulting string=w1303:string)  [unwired: 3 in, 1 out]
            n624 = call "SRV_SensorsQueue_Enqueue Element.vi"("error in (no error)"=w1306, "Data"=w1304, "Command"=w1303) -> ("error out"=w1305:errorcluster)  [unwired: 8 in]
          }
        }
      }
      frame "No Data" {
        n625 = Unbundle By Name(w1309) -> ("status"=w1313:bool, "code"=w1315:i32)
        n626 = call "SRV_Shutdown Flag.vi"("error in (no error)"=w1309) -> ("Shutdown Flag out"=w1307:bool, "error out"=w1310:errorcluster)  [unwired: 13 in]
        n627 = Equal?(x=w1315, y=1122 ("code (42: generic error)")) -> (x = y?=w1312:bool)
        n628 = Compound Arithmetic op=AND(w1313, w1312, w1307) -> (w1311:bool)
        n629 = case shown="True" w1311 {
          tunnel: w1310 -> [w1318 w1320]
          tunnel: [w1318 w1319] -> w1308
          frame False {
          }
          frame True {
            # "Shutting Down"
            n630 = call <vilib>:"Clear Errors.vi"("error in (no error)"=w1320) -> ("error out"=w1319:errorcluster)  [unwired: 5 in, 1 out]
          }
        }
      }
    }
    n631 = case shown="True" "Window Enabled?" {
      tunnel: w1196 -> [_ w1208]
      tunnel: w1195 -> [w1204 w1207]
      tunnel: w1194 -> [_ w1206]
      tunnel: [w1204 w1205] -> w1191
      frame False {
      }
      frame True {
        n632 = call "SRV_Update Replies Indicator.vi"("Replies ref"=w1206, "Text to Append"=w1208, "error in (no error)"=w1207) -> ("error out"=w1205:errorcluster)  [unwired: 11 in, 1 out]
      }
    }
    n633 = case shown="\"New PM\"" w1187 {
      tunnel: w1200 -> [w1210 w1211]
      tunnel: [w1209 w1211] -> w1199
      frame "Old" {
        n634 = call <vilib>:"Release Semaphore.vi"("semaphore"=w1210) -> ("semaphore out"=w1209:T23)  [unwired: 5 in, 1 out]
      }
      frame "New PM" {
      }
    }
    n635 = call "SRV_Manage Loop Errors.vi"("Loop Identifier"="Receive Action Loop", "error in (no error)"=w1191) -> ("error out"=w1190:errorcluster)  [unwired: 9 in]
    "i4" <- w1198
  }
  n636 = Unregister For Events(event registration refnum=w129, error in=w130) -> ()  [unwired: 1 out]
  n637 = Unbundle By Name(w127) -> ("Main Controller ref"=w114:refnum<vi>, "user event"=w126:refnum<user-event>)
  n638 = flat-sequence {
    tunnel: w139 -> [_]
    tunnel: w128 -> [_]
    tunnel: w126 -> [w1327]
    tunnel: [w1322] -> w147
    tunnel: w117 -> [w1321]
    tunnel: w109 -> [_]
    tunnel: w147 -> [_]
    tunnel: w114 -> [w1329]
    frame #0 {
      n639 = call "SRV_Generate User Exit Event.vi"("User Exit Event"=w1327) -> ("error out"=w1325:errorcluster, "User Exit Event out"=w1323:refnum<user-event>)  [unwired: 9 in]
      n640 = call "SRV_Wait (ms)+.vi"("milliseconds to wait"=u32 100 ("Delay (ms)"), "error in (no error)"=w1325) -> ("error out"=w1324:errorcluster)  [unwired: 12 in, 1 out]
      n641 = call <vilib>:"Release Semaphore Reference.vi"("semaphore"=w1321) -> ()  [unwired: 9 in, 2 out]
      n642 = Destroy User Event(user event=w1323, error in=w1324) -> (error out=w1322:errorcluster)
      "Status" <- ""
    }
    frame #1 {
      w1330 = FALSE  # Close When Done?
      # "Don't Close is the behavior desired by T Jump (Feb2014)"
      n643 = case shown="True" w1330 {
        tunnel: w1329 -> [_ w1331]
        frame False {
        }
        frame True {
          n644 = invoke class="VI" method="FP.Close"(reference=w1331) -> ()  [unwired: 2 in, 3 out]
        }
      }
    }
  }
